vi "UMLEditor_ReadXmiFile.vi"(1 "XmiFilePath":path=path "C:/Users/Mikael/Documents/EPA/ABC.xml", 5 "error in (no error)":errorcluster) -> (15 "classInfos":T14[](array[typedef]), 16 "TypeDefs":T10[](array[typedef]), 17 "Positions":cluster{"X":i32, "Y":i32}[](array[cluster]), 19 "error out":errorcluster)   [LabVIEW 2020]
doc: "Gets current diagram values"
uses:
  <resource>/Framework/Providers/Open_GDS/UML/ReversedEngineering/ReversedEngineering ClassInfoType.ctl
  <resource>/Framework/Providers/Open_GDS/ClassProviders/Common/CommonVIs/CommonVIs_VisibilityType.ctl
  <resource>/Framework/Providers/Open_GDS/ClassProviders/Common/CommonVIs/CommonVIs_AttributeInfoType.ctl
  <resource>/Framework/Providers/Open_GDS/ClassProviders/Common/CommonVIs/CommonVIs_AttributeDataType.ctl
  <resource>/Framework/Providers/Open_GDS/UML/ReversedEngineering/ReversedEngineering_ClassDependencyDetailsType.ctl
  <resource>/Framework/Providers/Open_GDS/ClassProviders/Common/ScriptingFunctions/SubVIs/Scripting_ViDependencyType.ctl
  <resource>/Framework/Providers/Open_GDS/UML/ReversedEngineering/ReversedEngineering TypeDefType.ctl
  <resource>/Framework/Providers/Open_GDS/UML/UMLEditor/UMLEditor_ReadXmiFile_Class.ctl
  <resource>/Framework/Providers/Open_GDS/UML/UMLEditor/UMLEditor_ReadXmiFile_Attribute.ctl
  <resource>/Framework/Providers/Open_GDS/UML/UMLEditor/UMLEditor_ReadXmiFile_Method.ctl
  <resource>/Framework/Providers/Open_GDS/UML/UMLEditor/UMLEditor_ReadXmiFile_DataTypes.ctl
  <resource>/Framework/Providers/Open_GDS/UML/UMLEditor/UMLEditor_ReadXmiFile_Association.ctl
  <resource>/Framework/Providers/Open_GDS/UML/UMLEditor/UMLEditor_ReadXmiFile_AssType.ctl
  <resource>/Framework/Providers/Open_GDS/UML/UMLEditor/UMLEditor_ReadXmiFile_Generalization.ctl
  <resource>/Framework/Providers/Open_GDS/UML/UMLEditor/UMLEditor_ReadXmiFile_Links.ctl
  <resource>/Framework/Providers/Open_GDS/UML/UMLEditor/UMLEditor_ReadXmiFile_LinkType.ctl
  <resource>/Framework/Providers/Open_GDS/ClassProviders/Common/CommonVIs/CommonVIs_ClassNamePathType.ctl
panel:
  out "ClassLinks":cluster{T1[]}[](array[cluster])
  out "ClassInheritance":cluster{"Genarilization":T3[]}[](array[cluster])
  out "Associations":T4[](array[typedef])
  out "Types":T6[](array[typedef])=[{"ID"="EAJava_float", "Name"="float"}, {"ID"="EAID_9D25F9E0_C95B_4aa1_AC76_B051C1862941", "Name"="A"}, {"ID"="EAID_C3DA8127_A723_4109_B2F4_88FBFDB77E9A", "Name"="C"}]
  out "ClassMethods":cluster{T7[]}[](array[cluster])=[{[{"ID"="EAID_5C196C86_2F09_4642_AF82_8C0E9349B8CC", "Name"="M1", "Visibility"=enum."public"}]}, {[{"ID"="EAID_F6ADC8AA_458B_42d5_92A7_EFF47D20A323", "Name"="M11", "Visibility"=enum."public"}]}, {[]}]
  out "ClassAttributes":cluster{T8[]}[](array[cluster])=[{[{"ID"="EAID_78A0901B_D286_47e2_BF0A_CBA2A3759587", "Name"="Att1", "Visibility"=enum."private", "RefIdType"="EAJava_float", "AssRefId"=""}]}, {[{"ID"="EAID_dst816E9D_1FF1_4b60_8E7A_E0ACE5709CF7", "Name"="", "Visibility"=enum."public", "RefIdType"="EAID_9D25F9E0_C95B_4aa1_AC76_B051C1862941", "AssRefId"="EAID_A6816E9D_1FF1_4b60_8E7A_E0ACE5709CF7"}, {"ID"="EAID_dst1490FC_8515_4843_A058_F8B338EB0930", "Name"="", "Visibility"=enum."public", "RefIdType"="EAID_C3DA8127_A723_4109_B2F4_88FBFDB77E9A", "AssRefId"="EAID_DE1490FC_8515_4843_A058_F8B338EB0930"}]}, {[]}]
  out "Classes":T9[](array[typedef])=[{"ID"="EAID_9D25F9E0_C95B_4aa1_AC76_B051C1862941", "Name"="A", "Visibility"=enum."public", "Stereotype"="", "Description"="", "X"=0, "Y"=0}, {"ID"="EAID_C026E737_BCF9_4d6d_B726_90C39C0C8268", "Name"="B", "Visibility"=enum."public", "Stereotype"="", "Description"="", "X"=0, "Y"=0}, {"ID"="EAID_C3DA8127_A723_4109_B2F4_88FBFDB77E9A", "Name"="C", "Visibility"=enum."public", "Stereotype"="", "Description"="", "X"=0, "Y"=0}]
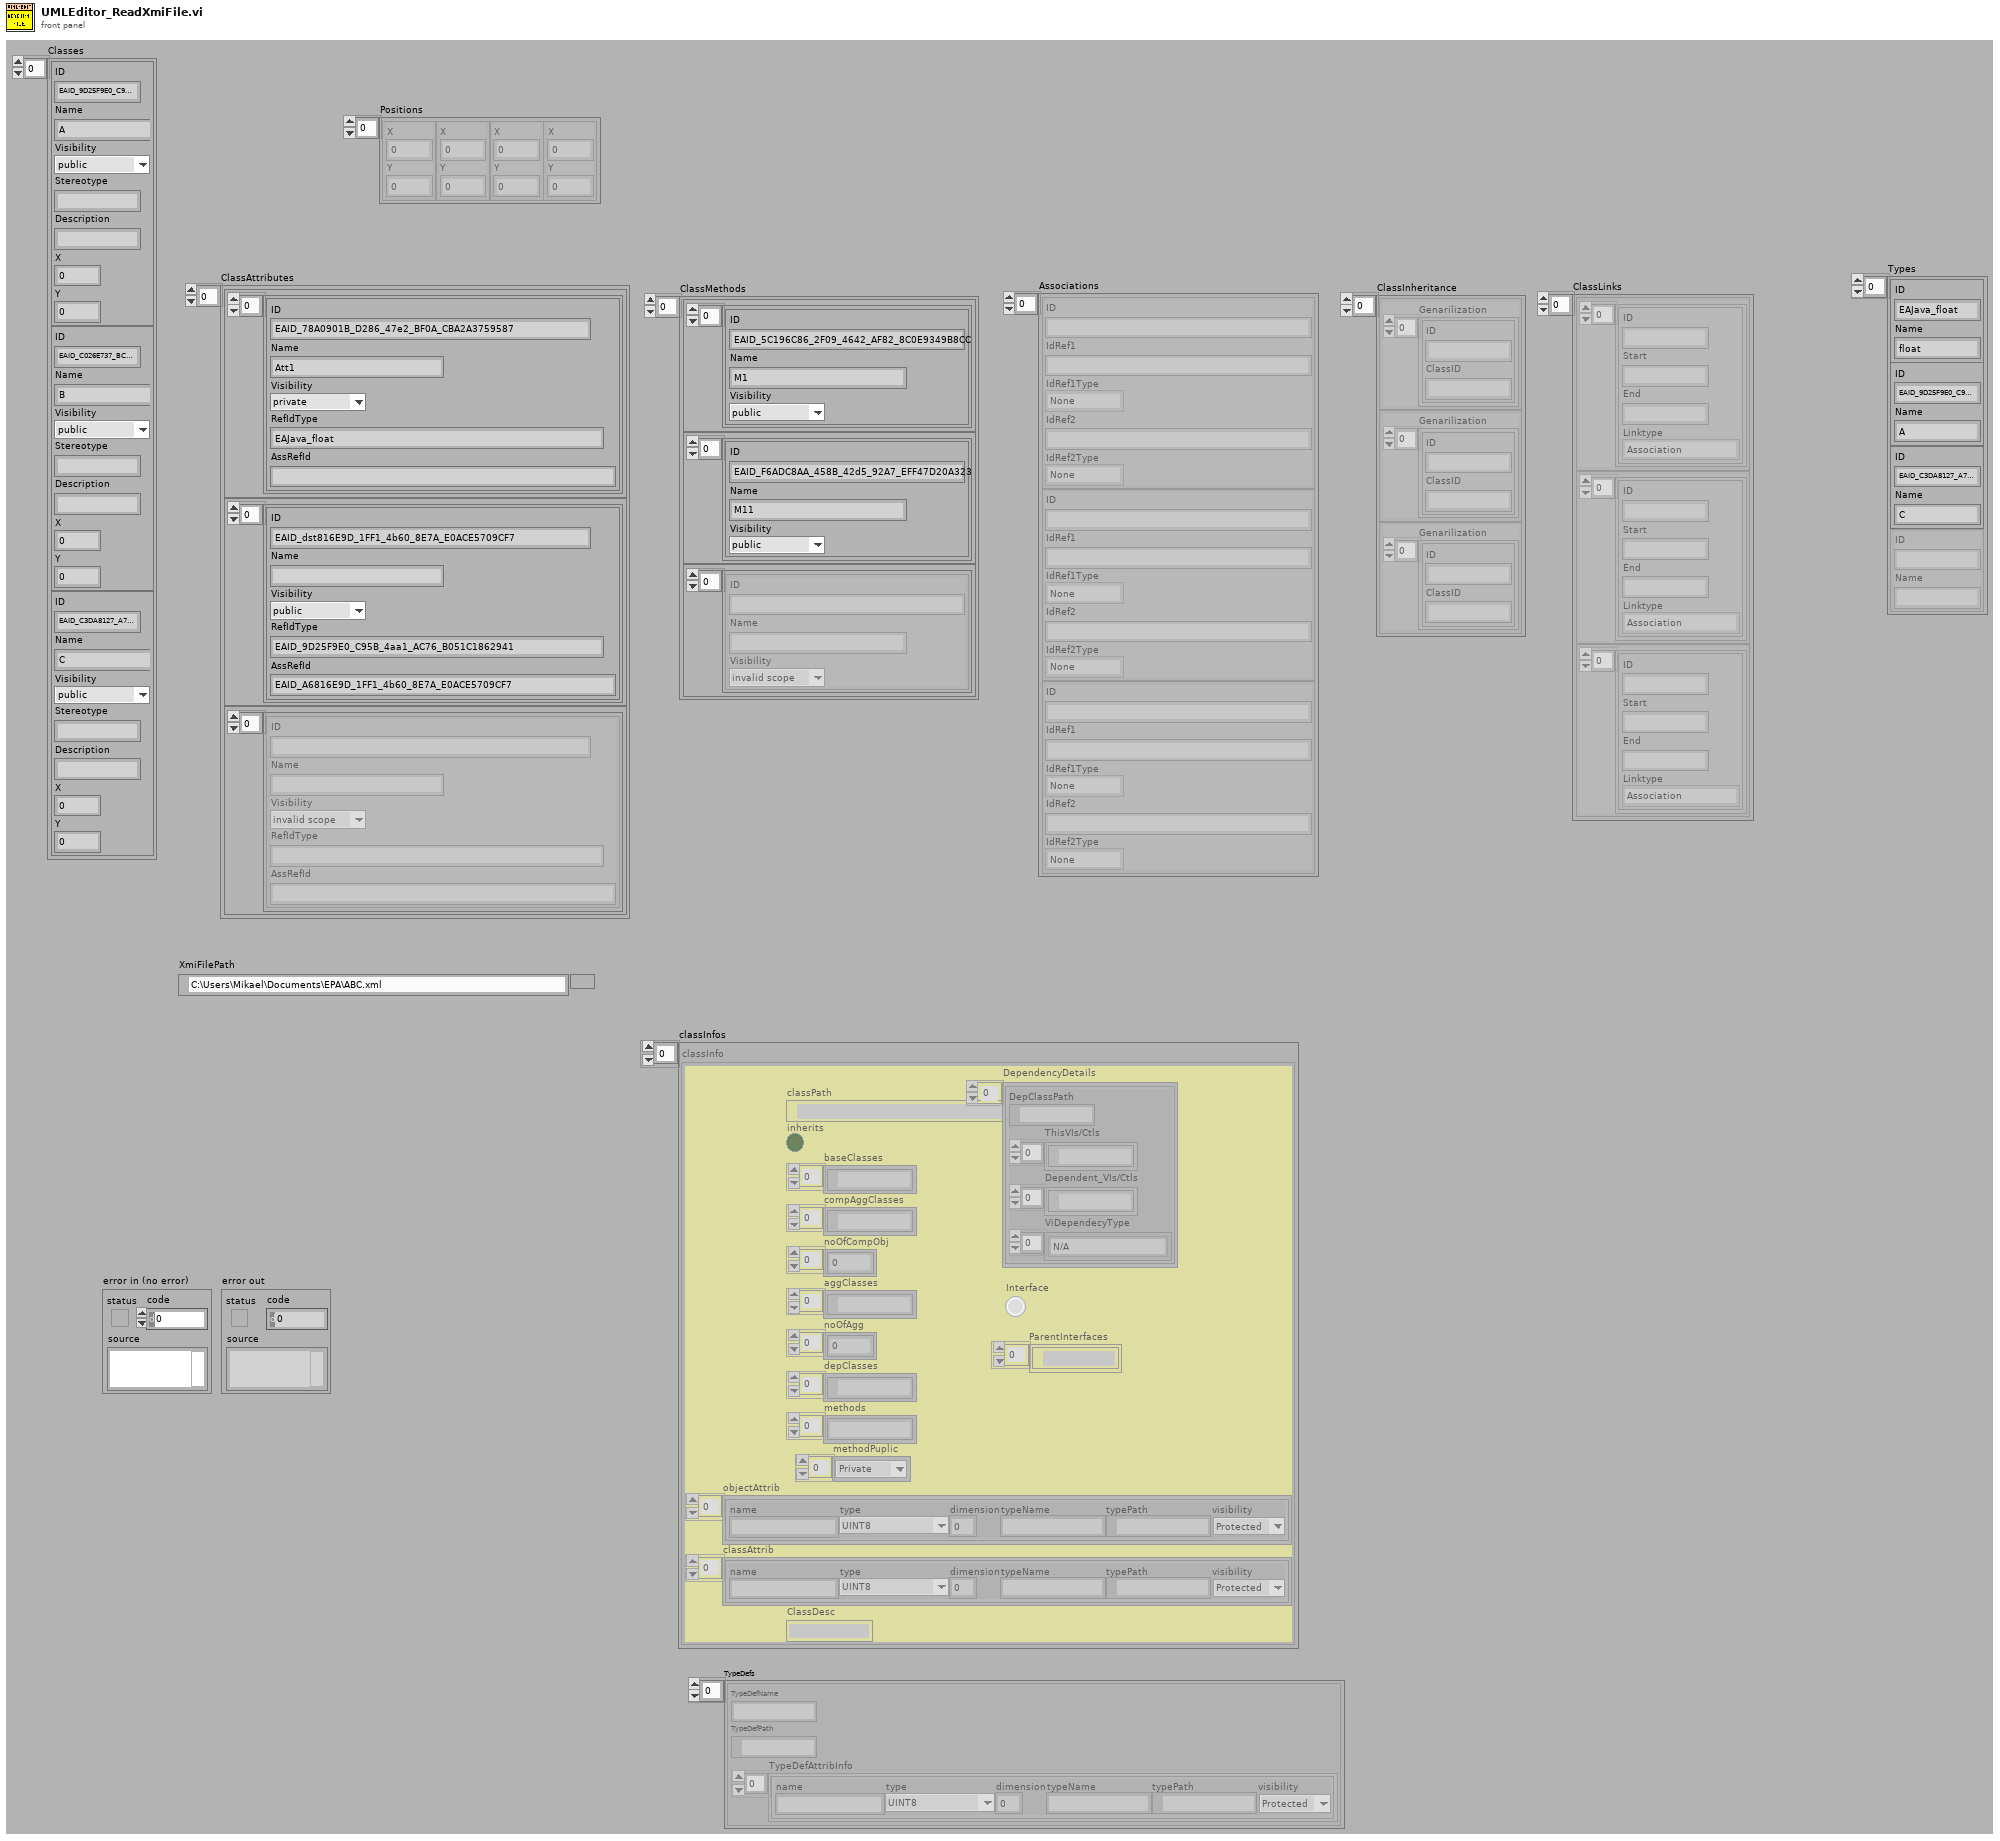
[diagram p1: front panel]
types:
  T1 = typedef "UMLEditor_ReadXmiFile_Links.ctl" = cluster{"ID":string, "Start":string, "End":string, "Linktype":T2}
  T2 = typedef "UMLEditor_ReadXmiFile_LinkType.ctl" = enum16{"Association", "Aggregation", "Generalization"}
  T3 = typedef "UMLEditor_ReadXmiFile_Generalization.ctl" = cluster{"ID":string, "ClassID":string}
  T4 = typedef "UMLEditor_ReadXmiFile_Association.ctl" = cluster{"ID":string, "IdRef1":string, "IdRef1Type":T5, "IdRef2":string, "IdRef2Type":T5}
  T5 = typedef "UMLEditor_ReadXmiFile_AssType.ctl" = enum16{"None", "Shared", "Composite"}
  T6 = typedef "UMLEditor_ReadXmiFile_DataTypes.ctl" = cluster{"ID":string, "Name":string}
  T7 = typedef "UMLEditor_ReadXmiFile_Method.ctl" = cluster{"ID":string, "Name":string, "Visibility":enum32{"invalid scope", "public", "private", "protected", "community"}}
  T8 = typedef "UMLEditor_ReadXmiFile_Attribute.ctl" = cluster{"ID":string, "Name":string, "Visibility":enum32{"invalid scope", "public", "private", "protected", "community"}, "RefIdType":string, "AssRefId":string}
  T9 = typedef "UMLEditor_ReadXmiFile_Class.ctl" = cluster{"ID":string, "Name":string, "Visibility":enum32{"invalid scope", "public", "private", "protected", "community"}, "Stereotype":string, "Description":string, "X":i32, "Y":i32}
  T10 = typedef "ReversedEngineering TypeDefType.ctl" = cluster{"TypeDefName":string, "TypeDefPath":path, "TypeDefAttribInfo":T11[]}
  T11 = typedef "CommonVIs_AttributeInfoType.ctl" = cluster{"name":string, "type":T12, "dimension":i32, "typeName":string, "typePath":path, "visibility":T13}
  T12 = typedef "CommonVIs_AttributeDataType.ctl" = enum16{"UINT8", "INT8", "UINT16", "INT16", "UINT32", "INT32", "UINT64", "INT64", "SGL", "DBL", "EXT", "CSG", "CDB", "CXT", "TimeStamp", "STRING", "PATH", "BOOL", "ENUM", "RefNum", "VIRefNum", "LabVIEW Class", "Cluster", "Variant", "TypeDef", "Waveform", "LabVIEW Object", "Other", "void", "Set", "Map"}
  T13 = typedef "CommonVIs_VisibilityType.ctl" = enum16{"Public", "Private", "Protected"}
  T14 = typedef "ReversedEngineering ClassInfoType.ctl" = cluster{"classPath":path, "inherits":bool, "baseClasses":path[], "compAggClasses":path[], "noOfCompObj":i32[], "aggClasses":path[], "noOfAgg":i32[], "depClasses":path[], "methods":string[], "methodPuplic":T13[], "objectAttrib":T11[], "classAttrib":T11[], "ClassDesc":string, "DependencyDetails":T15[], "Interface":bool, "ParentInterfaces":path[]}
  T15 = typedef "ReversedEngineering_ClassDependencyDetailsType.ctl" = cluster{"DepClassPath":path, "ThisVIs/Ctls":path[], "Dependent_VIs/Ctls":path[], "ViDependecyType":T16[]}
  T16 = typedef "Scripting_ViDependencyType.ctl" = enum16{"N/A", "Launches"}
  T17 = cluster{"dependencyClassPath":path[], "topVIPath":path, "classInfos":T14[], "calleesVIs":path[], "VIRef":refnum<vi>[], "TypeDefs":T10[], "TopVIPath":path, "SearchOnlyClasses":bool, "SearchDirs":path[], "SearchOnlyTopVIs":bool, "lvclasses":path[], "Classes":T9[], "ClasseStrings":string[], "ClassAttributes":cluster{T8[]}[], "ClassMethods":cluster{T7[]}[], "text":string, "Types":T6[], "ClassInheritance":cluster{"Genarilization":T3[]}[], "Associations":T4[], "Positions":cluster{"X":i32, "Y":i32}[], "ClassLinks":cluster{T1[]}[]}
  T18 = enum32{"invalid scope", "public", "private", "protected", "community"}
  T19 = typedef "CommonVIs_ClassNamePathType.ctl" = cluster{"ClassNamn":string, "ClassPath":path, "InterfaceClass":bool}
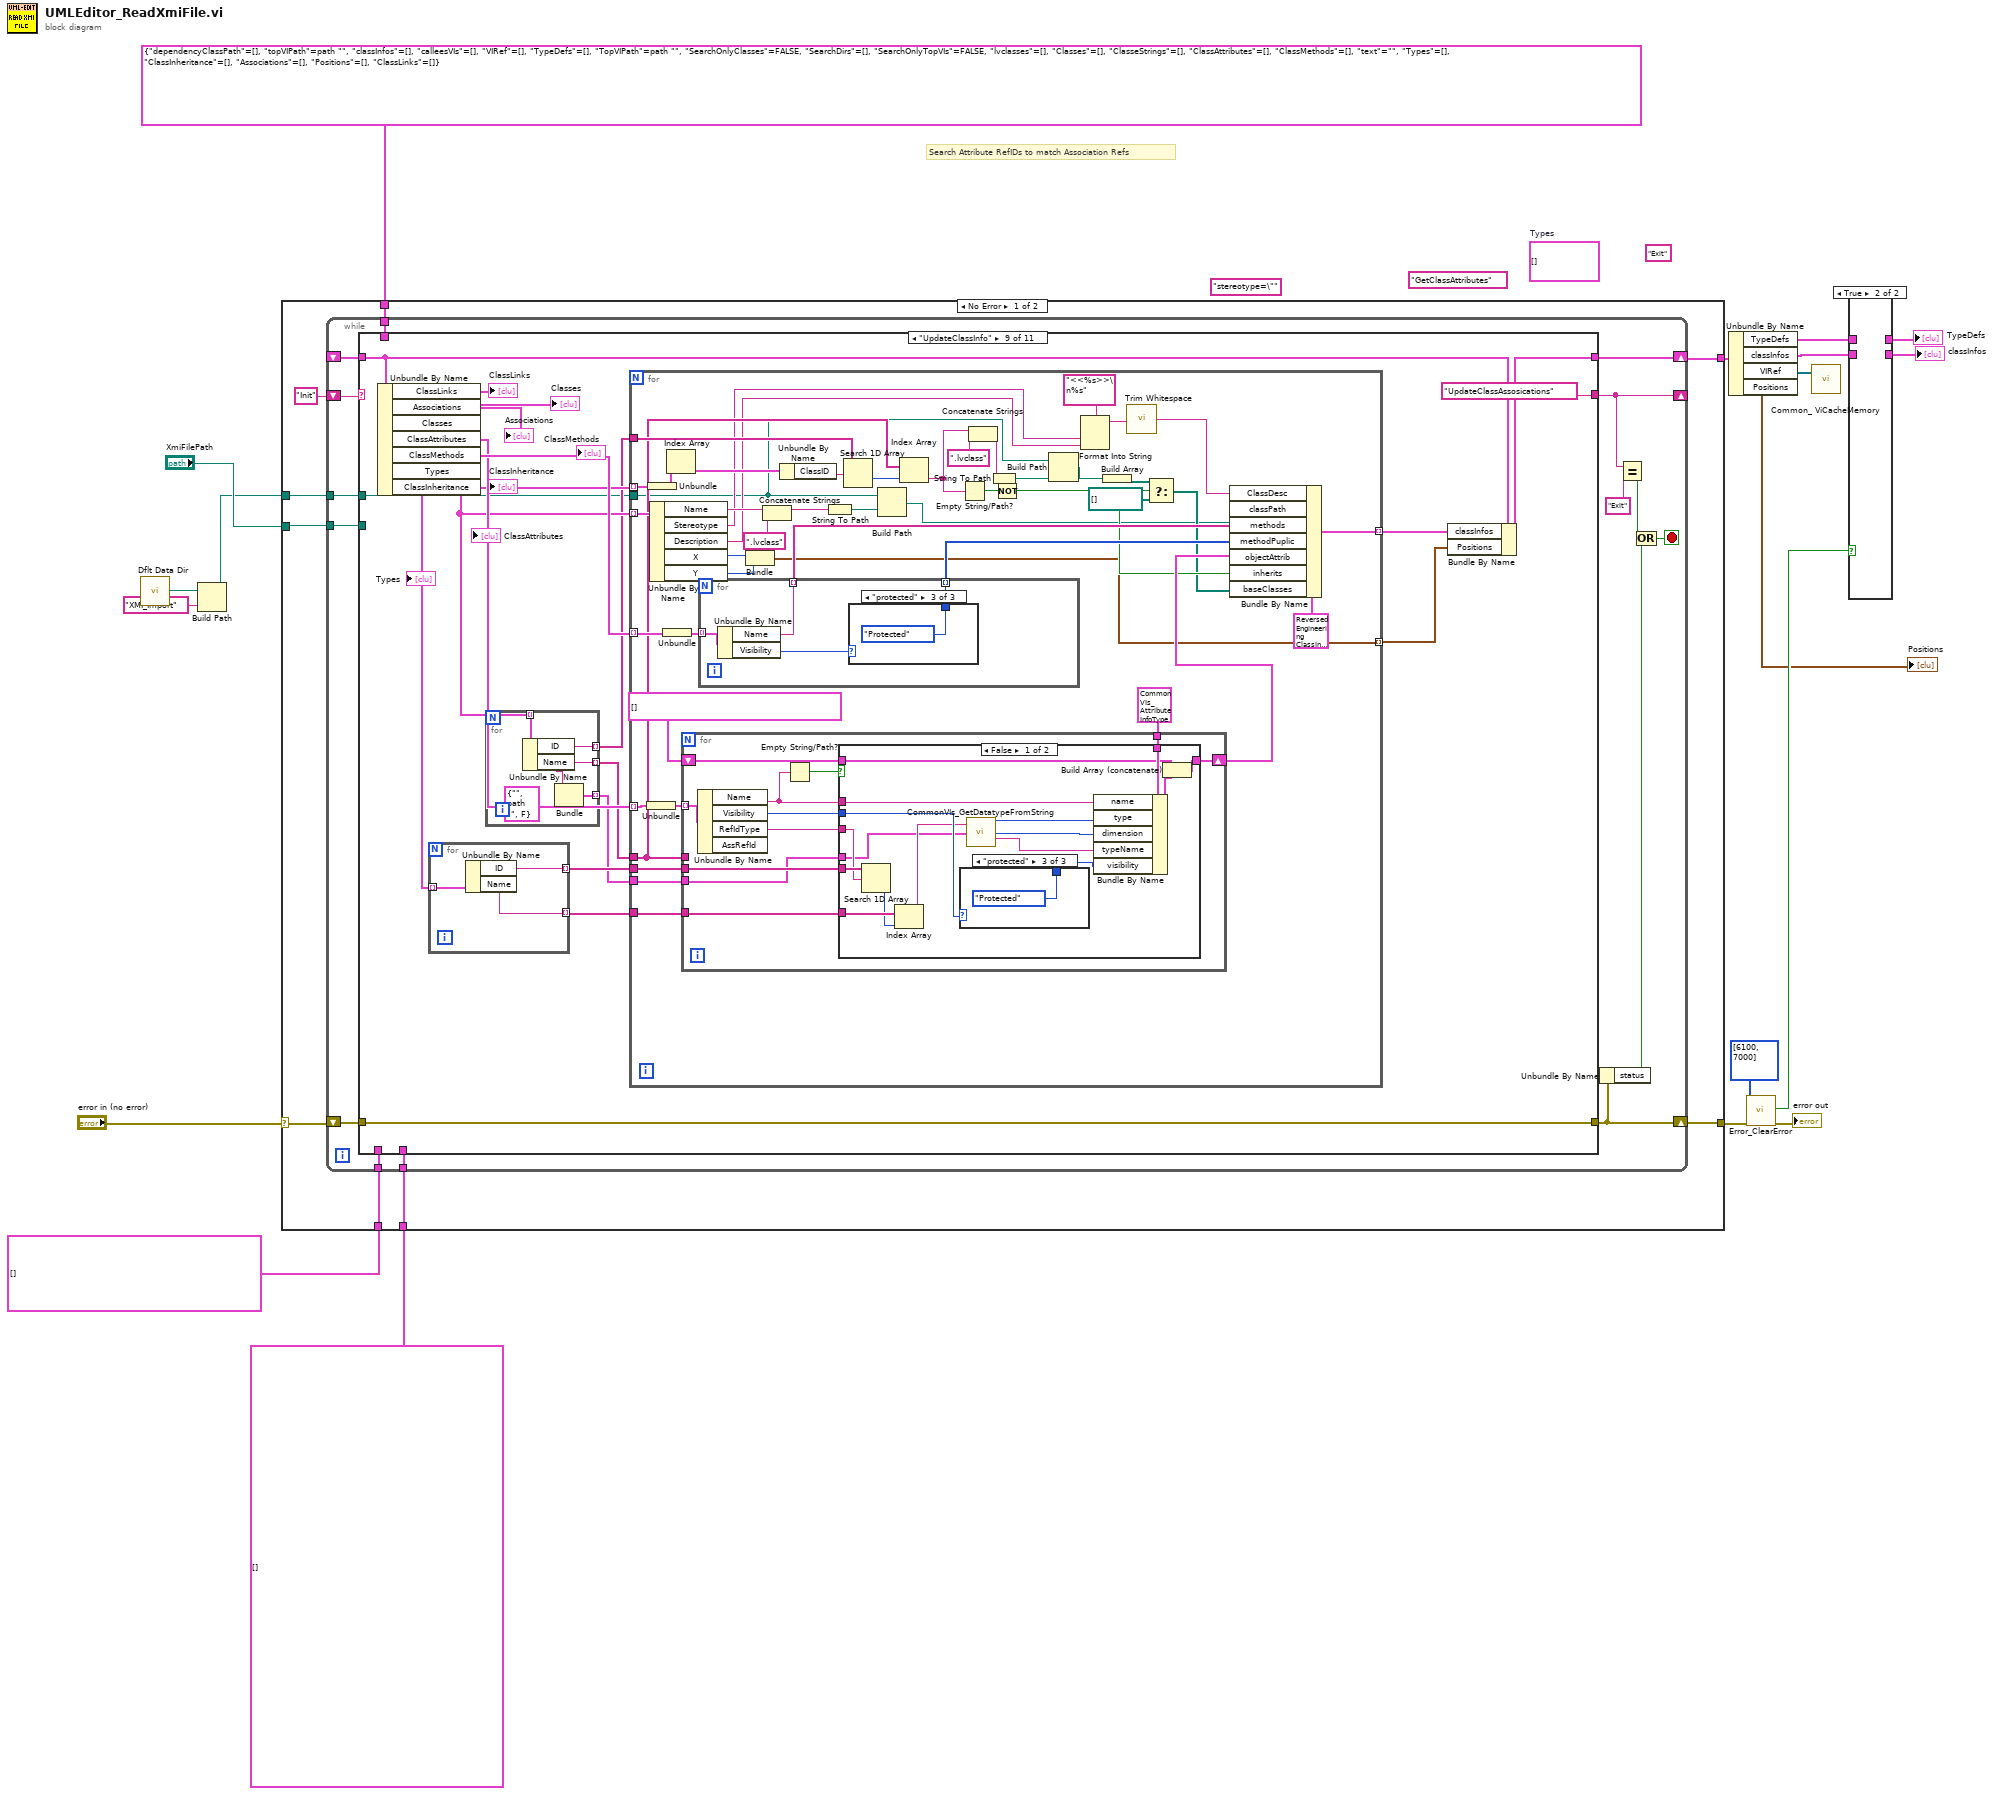
[diagram p0: block diagram]
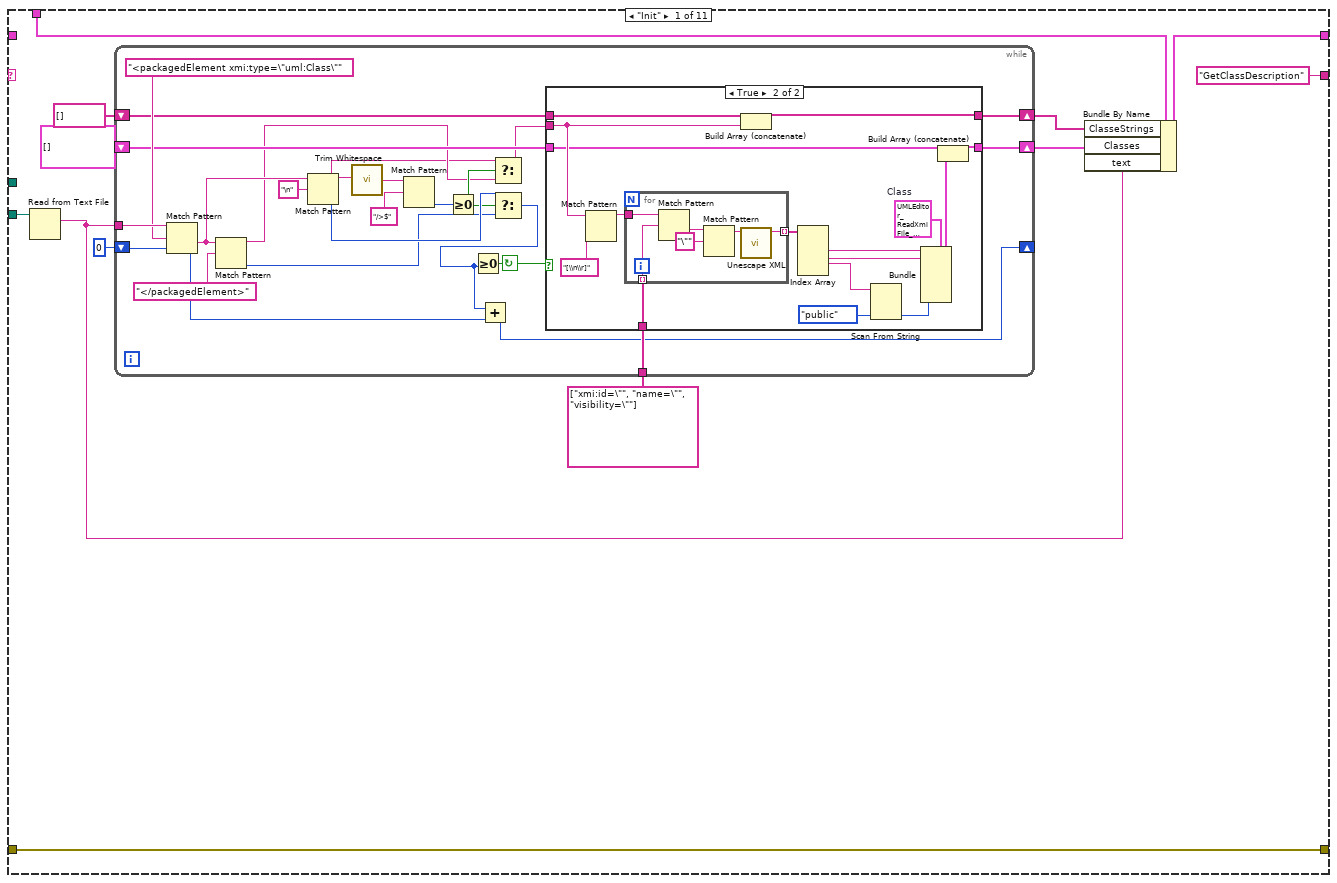
[diagram p3: hidden frame]
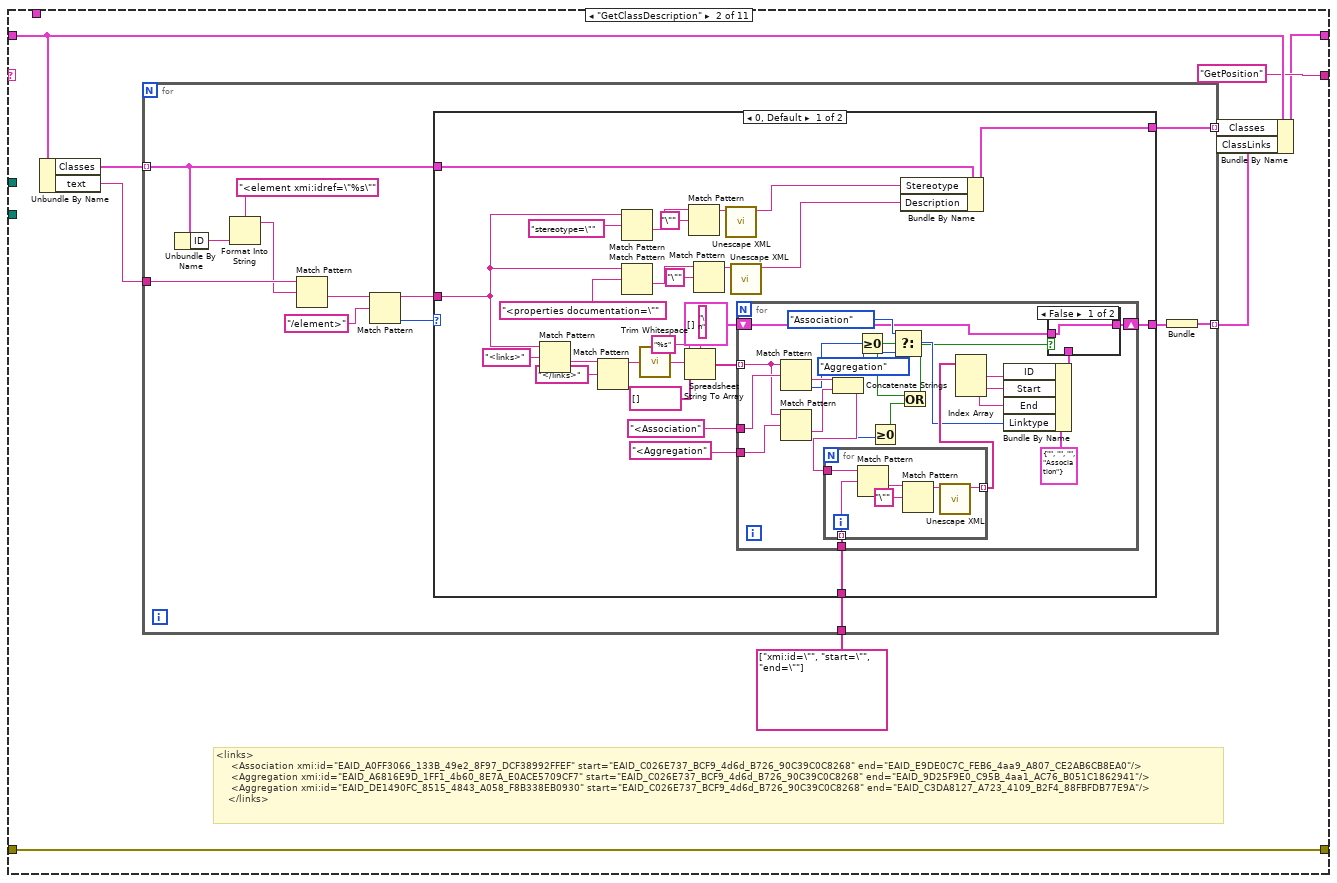
[diagram p5: hidden frame]
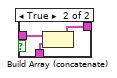
[diagram p6: hidden frame]
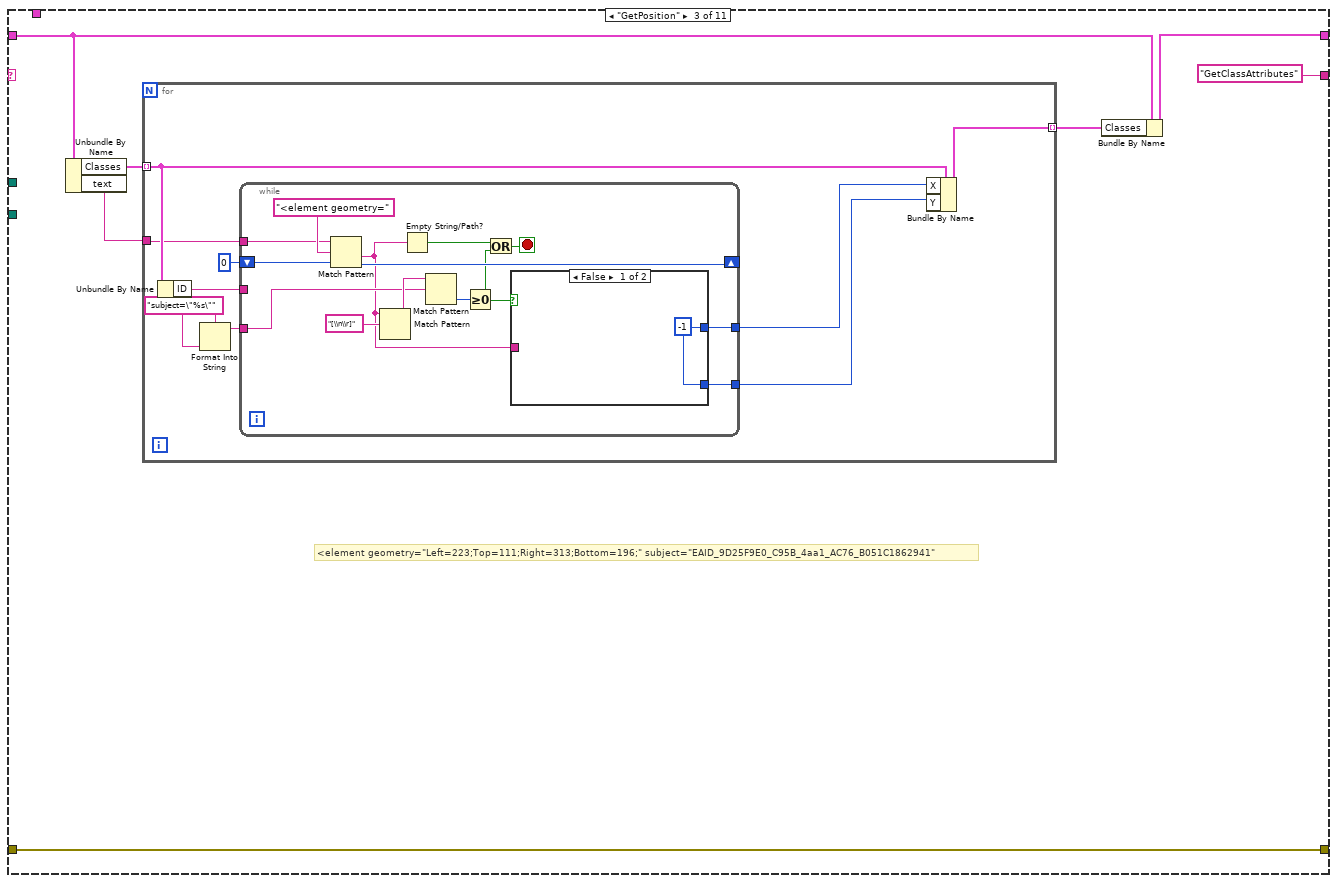
[diagram p8: hidden frame]
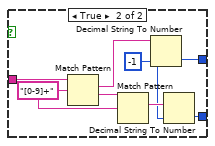
[diagram p9: hidden frame]
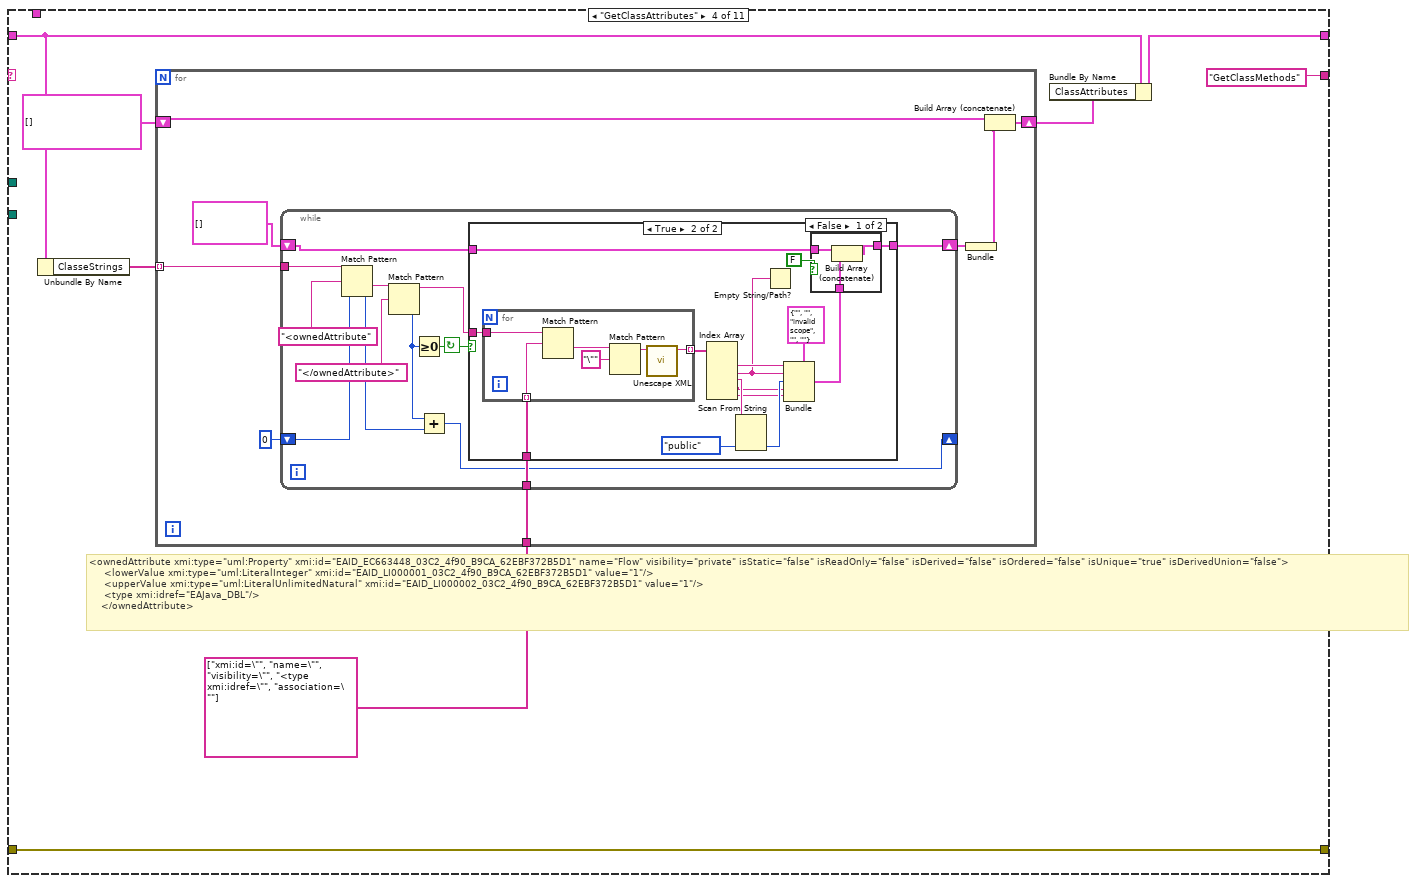
[diagram p10: hidden frame]
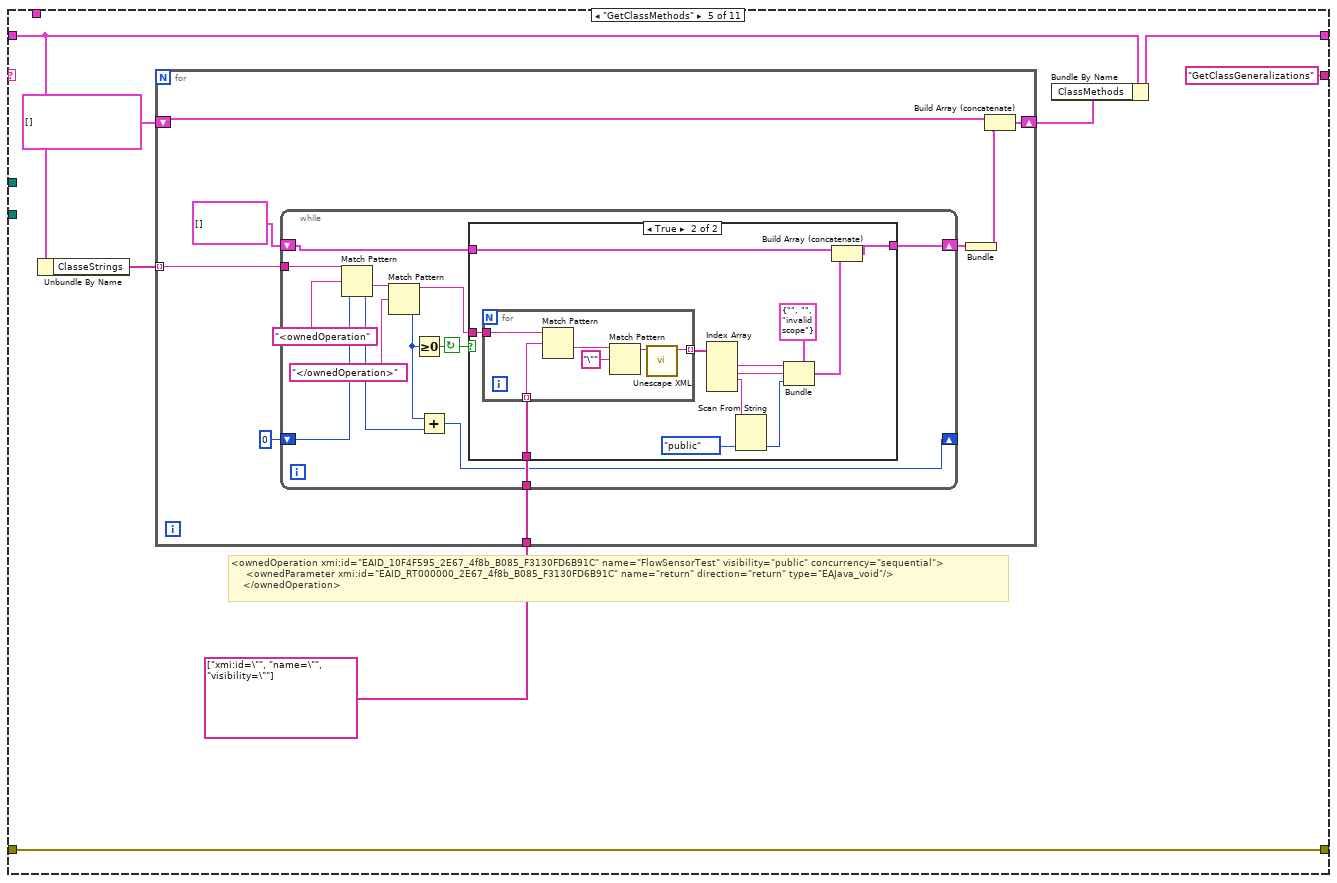
[diagram p13: hidden frame]
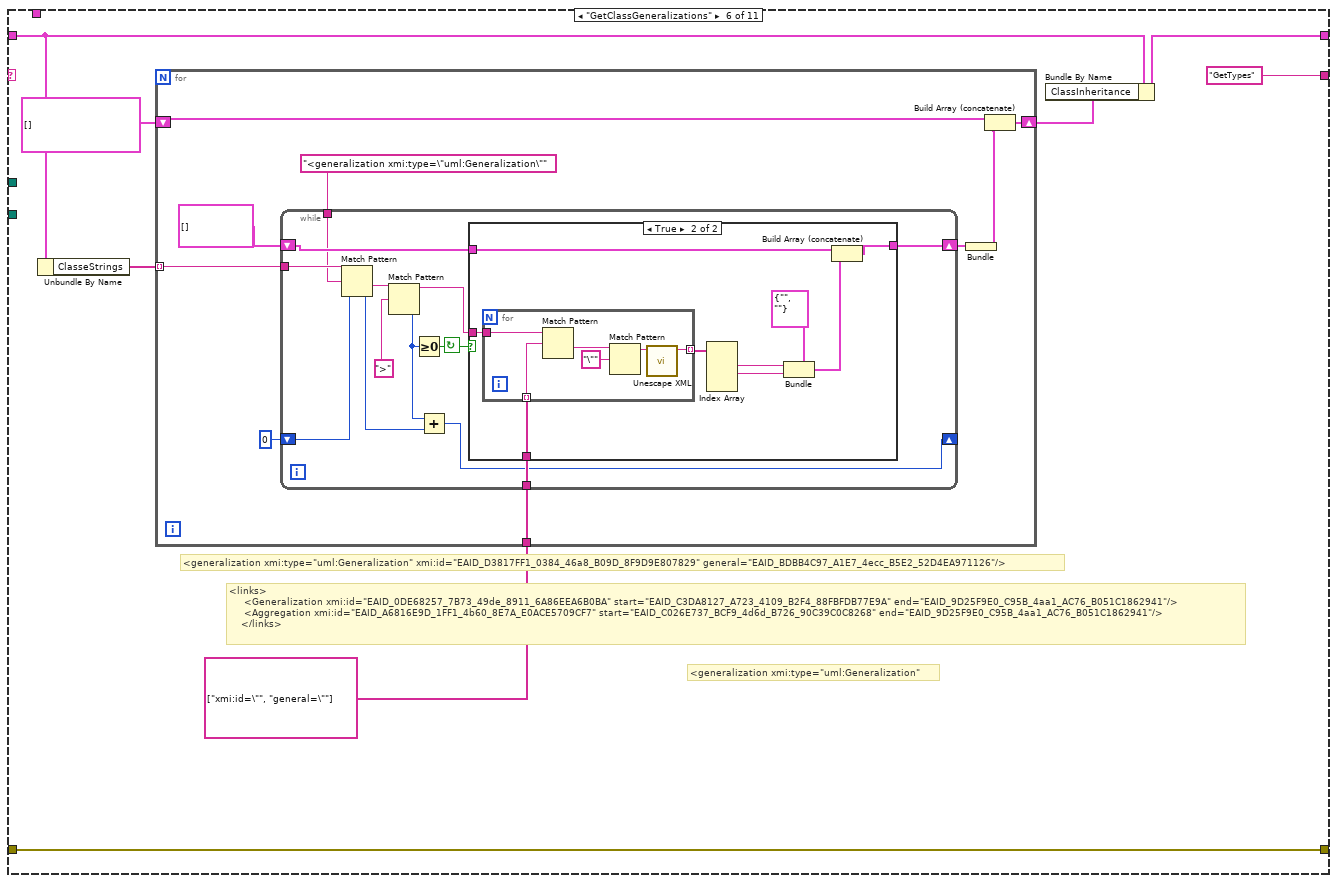
[diagram p15: hidden frame]
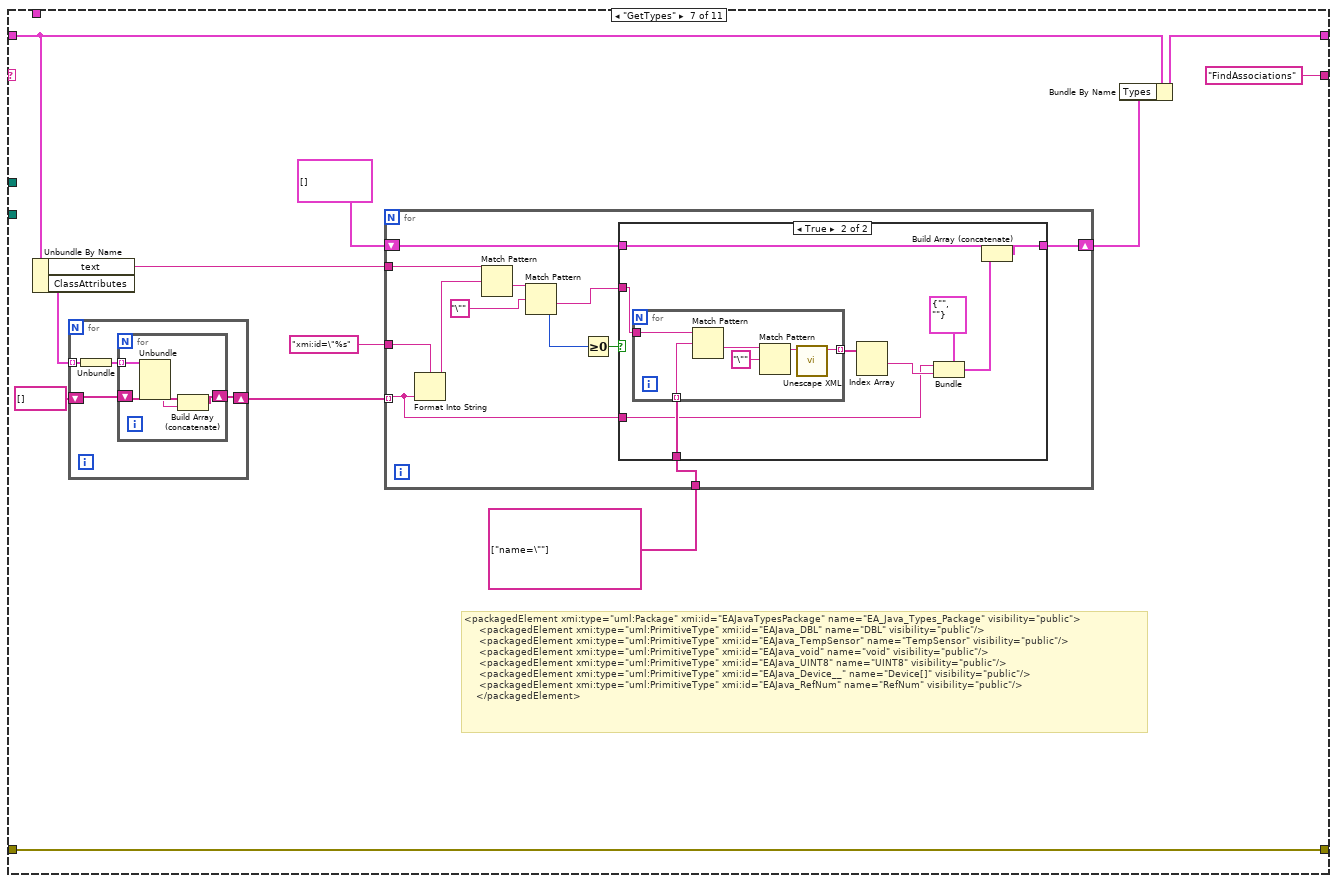
[diagram p17: hidden frame]
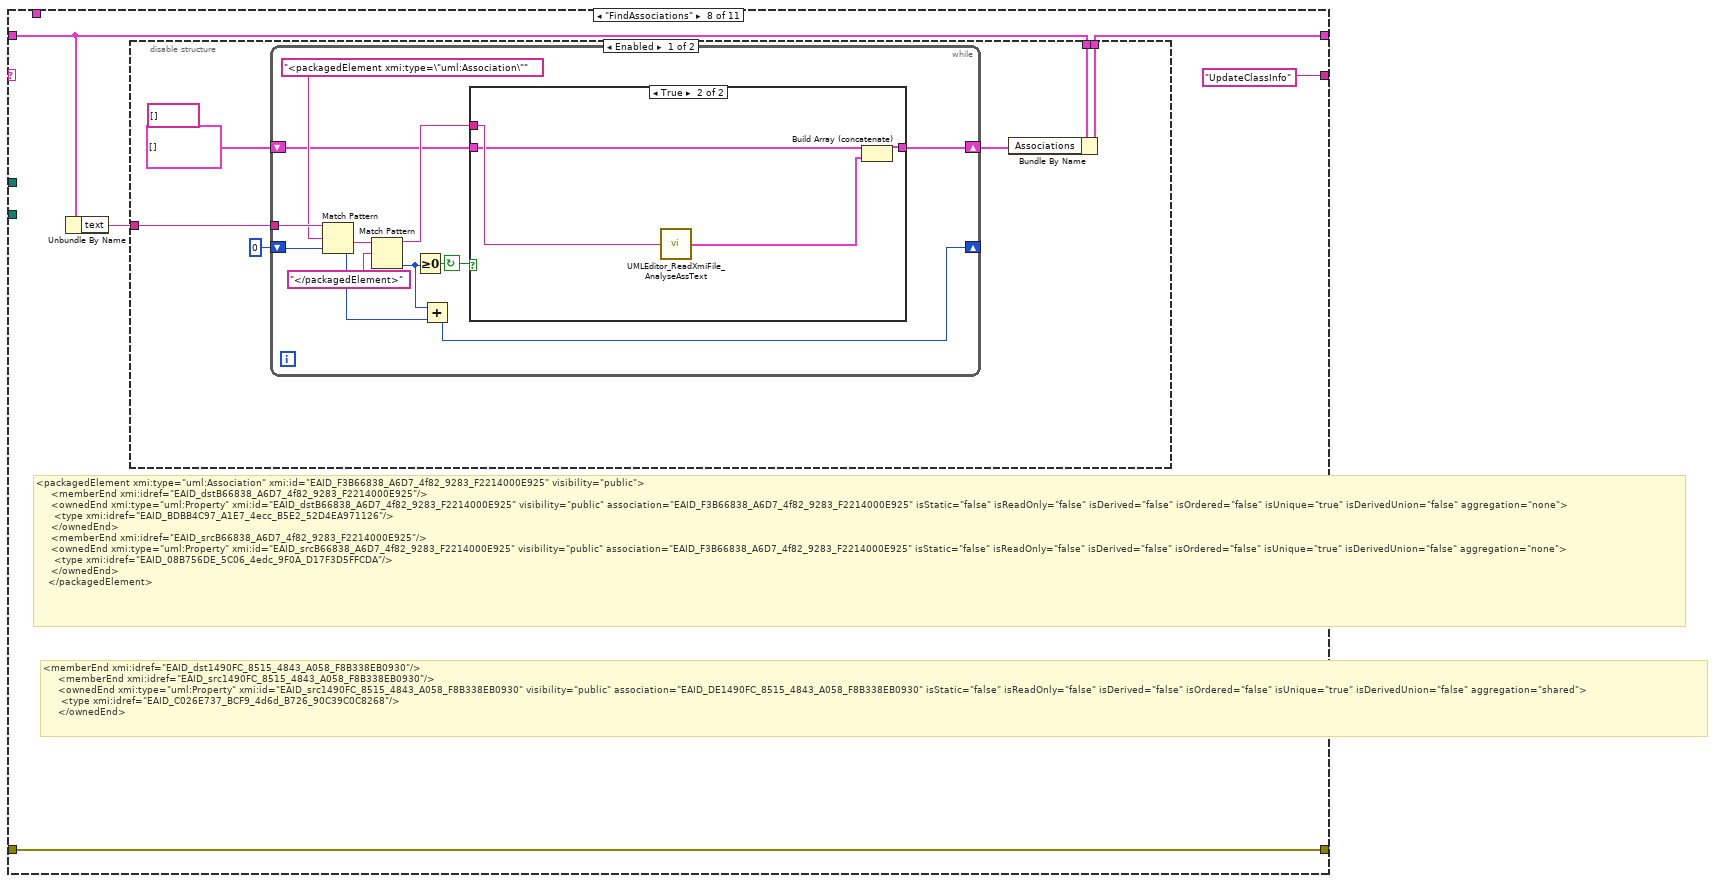
[diagram p19: hidden frame]
diagram:
  (unwired) "Exit" ("y")
  (unwired) "GetClassAttributes"
  (unwired) "stereotype=\""
  (unwired) T6[] []  # Types
  # "Search Attribute RefIDs to match Association Refs"
  n1 = call <vilib>:"Dflt Data Dir.vi"() -> ("App:Default Data Directory"=w3:path)
  n2 = Build Path(base path=w3, name or relative path="XMI_Import") -> (appended path=w1:path)
  n3 = case shown="No Error" "error in (no error)" {
    selector: "error in (no error)" -> [w27 w747]
    tunnel: [w26 w747] -> w16
    tunnel: [w25 _] -> w18
    tunnel: T17 {"dependencyClassPath"=[], "topVIPath"=path "", "classInfos"=[], "calleesVIs"=[], "VIRef"=[], "TypeDefs"=[], "TopVIPath"=path "", "SearchOnlyClasses"=FALSE, "SearchDirs"=[], "SearchOnlyTopVIs"=FALSE, "lvclasses"=[], "Classes"=[], "ClasseStrings"=[], "ClassAttributes"=[], "ClassMethods"=[], "text"="", "Types"=[], "ClassInheritance"=[], "Associations"=[], "Positions"=[], "ClassLinks"=[]} ("Cluster") -> [w24 _]
    tunnel: T14[] [] -> [w23 _]
    tunnel: T10[] [] -> [w22 _]
    tunnel: "XmiFilePath" -> [w21 _]
    tunnel: w1 -> [w20 _]
    frame No Error {
      n4 = while {
        shift-right: [w40] -> _
        shift-left: "Init" -> [w43]
        shift-right: [w41] -> w26
        shift-left: w27 -> [w42]
        shift-right: [w34] -> w25
        shift-left: _ -> [w35]
        tunnel: w24 -> [w33]
        tunnel: w23 -> [w32]
        tunnel: w22 -> [w31]
        tunnel: w21 -> [w30]
        tunnel: w20 -> [w29]
        stop <- w36 stop-if-true
        n5 = case shown="\"UpdateClassInfo\"" w43 {
          tunnel: w42 -> [w55 w106 w187 w227 w281 w329 w375 w427 w469 w568 w744]
          tunnel: [w55 w106 w187 w227 w281 w329 w375 w427 w469 w568 w744] -> w41
          tunnel: ["GetClassDescription" "GetPosition" "GetClassAttributes" "GetClassMethods" "GetClassGeneralizations" "GetTypes" "FindAssociations" "UpdateClassInfo" "UpdateClassAssosications" ("y") "Exit" ("y") "Exit" ("y")] -> w40
          tunnel: w35 -> [_ w111 w192 w230 w285 w333 w384 w423 w461 w564 w746]
          tunnel: [w46 w109 w190 w228 w283 w331 w383 w426 w460 w575 w746] -> w34
          tunnel: w33 -> [w47 _ _ _ _ _ _ _ _ _ _]
          tunnel: w32 -> [_ _ _ _ _ _ _ _ _ _ _]
          tunnel: w31 -> [_ _ _ _ _ _ _ _ _ _ _]
          tunnel: w30 -> [w54 _ _ _ _ _ _ _ _ _ _]
          tunnel: w29 -> [_ _ _ _ _ _ _ _ w454 w569 _]
          frame "Init" {
            n6 = Read from Text File(file (use dialog)=w54) -> (text=w45:string)  [unwired: 3 in, 3 out]
            n7 = while {
              tunnel: w45 -> [w79]
              shift-right: [w75] -> w48
              shift-left: string[] [] -> [w76]
              shift-right: [w68] -> _
              shift-left: 0 ("offset past match") -> [w73]
              tunnel: string[] ["xmi:id=\"", "name=\"", "visibility=\""] -> [w72]
              shift-right: [w71] -> w49
              shift-left: T9[] [] -> [w70]
              stop <- w74 continue-if-true
              n8 = Match Pattern(string=w79, regular expression="<packagedElement xmi:type=\"uml:Class\"", offset (0)=w73) -> (after substring=w62:string, offset past match=w69:i32)  [unwired: 2 out]
              n9 = Match Pattern(string=w62, regular expression="</packagedElement>") -> (before substring=w58:string, offset past match=w60:i32)  [unwired: 1 in, 2 out]
              n10 = Match Pattern(string=w62, regular expression="\n") -> (before substring=w57:string, offset past match=w67:i32)  [unwired: 1 in, 2 out]
              n11 = call <vilib>:"Trim Whitespace.vi"("string"=w57) -> ("trimmed string"=w64:string)  [unwired: 1 in]
              n12 = Match Pattern(string=w64, regular expression="/>$") -> (offset past match=w66:i32)  [unwired: 1 in, 3 out]
              n13 = Greater Or Equal To 0?(x=w66) -> (x >= 0?=w59:bool)
              n14 = Select(t=w57, s=w59, f=w58) -> (s? t:f=w56:string)
              n15 = Select(t=w67, s=w59, f=w60) -> (s? t:f=w61:i32)
              n16 = Greater Or Equal To 0?(x=w61) -> (x >= 0?=w74:bool)
              n17 = Add(x=w61, y=w69) -> (x+y=w68:i32)
              n18 = case shown="True" w74 {
                tunnel: w76 -> [w81 w97]
                tunnel: [w81 w96] -> w75
                tunnel: w56 -> [_ w95]
                tunnel: w72 -> [_ w93]
                tunnel: w70 -> [w80 w83]
                tunnel: [w80 w84] -> w71
                frame False {
                }
                frame True {
                  w90 = T9 {"ID"="", "Name"="", "Visibility"=enum."invalid scope", "Stereotype"="", "Description"="", "X"=0, "Y"=0}  # Class
                  n19 = Match Pattern(string=w95, regular expression="[\\n\\r]") -> (before substring=w92:string)  [unwired: 1 in, 3 out]
                  n20 = for {
                    tunnel: w93 -> [w103] mode=indexing
                    tunnel: w92 -> [w102]
                    tunnel: [w98] -> w91 mode=indexing
                    n21 = Match Pattern(string=w102, regular expression=w103) -> (after substring=w101:string)  [unwired: 1 in, 3 out]
                    n22 = Match Pattern(string=w101, regular expression="\"") -> (before substring=w99:string)  [unwired: 1 in, 3 out]
                    n23 = call <vilib>:"Unescape XML.vi"("XML String In"=w99) -> ("XML String Out"=w98:string)  [unwired: 9 in, 1 out]
                  }
                  n24 = Build Array (concatenate)(w97, w95) -> (w96:string[])
                  n25 = Index Array(array=w91) -> (element #1=w89:string, element #2=w88:string, element #3=w87:string)  [unwired: 4 in, 1 out]
                  n26 = Scan From String(input string=w87, default 1=T18."public" ("Visibility")) -> (output 1=w86:T18)  [unwired: 3 in, 3 out]
                  n27 = Bundle(cluster=w90, "ID"=w89, "Name"=w88, "Visibility"=w86) -> (w82:T9)  [unwired: 4 in]
                  n28 = Build Array (concatenate)(w83, w82) -> (w84:T9[])
                }
              }
            }
            n29 = Bundle By Name(cluster=w47, "ClasseStrings"=w48, "Classes"=w49, "text"=w45) -> (w46:T17)
          }
          frame "GetClassDescription" {
            # "<links>\n\t\t\t\t\t<Association xmi:id=\"EAID_A0FF3066_133B_49e2_8F97_DCF38992FFEF\" start=\"EAID_C026E737_BCF9_4d6d_B726_90C39C0C8268\" end=\"EAID_E9DE0C7C_FEB6_4aa9_A807_CE2AB6CB8EA0\"/>\n\t\t\t\t\t<Aggregation xmi:id=\"EAID_A6816E9D_1FF1_4b60_8E7A_E0ACE5709CF7\" start=\"EAID_C026E737_BCF9_4d6d_B726_90C39C0C8268\" end=\"EAID_9D25F9E0_C95B_4aa1_AC76_B051C1862941\"/>\n\t\t\t\t\t<Aggregation xmi:id=\"EAID_DE1490FC_8515_4843_A058_F8B338EB0930\" start=\"EAID_C026E737_BCF9_4d6d_B726_90C39C0C8268\" end=\"EAID_C3DA8127_A723_4109_B2F4_88FBFDB77E9A\"/>\n\t\t\t\t</links>"
            n30 = Unbundle By Name(w111) -> ("Classes"=w112:T9[], "text"=w107:string)
            n31 = for {
              tunnel: w112 -> [w123] mode=indexing
              tunnel: [w125] -> w108 mode=indexing
              tunnel: w107 -> [w121]
              tunnel: string[] ["xmi:id=\"", "start=\"", "end=\""] -> [w115]
              tunnel: [w113] -> w104 mode=indexing
              n32 = Unbundle By Name(w123) -> ("ID"=w122:string)
              n33 = Format Into String(format string="<element xmi:idref=\"%s\"", w122) -> (resulting string=w120:string)  [unwired: 2 in, 1 out]
              n34 = Match Pattern(string=w121, regular expression=w120) -> (after substring=w119:string)  [unwired: 1 in, 3 out]
              n35 = Match Pattern(string=w119, regular expression="/element>") -> (before substring=w116:string, offset past match=w117:i32)  [unwired: 1 in, 2 out]
              n36 = case shown="0, Default" w117 {
                tunnel: [w152 w186] -> w125
                tunnel: w123 -> [w151 w186]
                tunnel: w116 -> [w140 _]
                tunnel: w115 -> [w128 _]
                tunnel: [w126 _] -> w114
                frame 0, Default {
                  n37 = Match Pattern(string=w140, regular expression="<links>") -> (after substring=w138:string)  [unwired: 1 in, 3 out]
                  n38 = Match Pattern(string=w138, regular expression="</links>") -> (before substring=w136:string)  [unwired: 1 in, 3 out]
                  n39 = Match Pattern(string=w140, regular expression="stereotype=\"") -> (after substring=w142:string)  [unwired: 1 in, 3 out]
                  n40 = Match Pattern(string=w140, regular expression="<properties documentation=\"") -> (after substring=w147:string)  [unwired: 1 in, 3 out]
                  n41 = call <vilib>:"Trim Whitespace.vi"("string"=w136) -> ("trimmed string"=w135:string)  [unwired: 1 in]
                  n42 = Spreadsheet String To Array(delimiter (Tab)="\n", format string="%s", spreadsheet string=w135, array type (2D Dbl)=string[] []) -> (array=w131:string[])
                  n43 = Match Pattern(string=w142, regular expression="\"") -> (before substring=w144:string)  [unwired: 1 in, 3 out]
                  n44 = Match Pattern(string=w147, regular expression="\"") -> (before substring=w148:string)  [unwired: 1 in, 3 out]
                  n45 = call <vilib>:"Unescape XML.vi"("XML String In"=w144) -> ("XML String Out"=w141:string)  [unwired: 9 in, 1 out]
                  n46 = call <vilib>:"Unescape XML.vi"("XML String In"=w148) -> ("XML String Out"=w146:string)  [unwired: 9 in, 1 out]
                  n47 = for {
                    tunnel: w131 -> [w174] mode=indexing
                    tunnel: "<Association" ("regular expression") -> [w175]
                    tunnel: "<Aggregation" ("regular expression") -> [w173]
                    tunnel: w128 -> [w169]
                    shift-right: [w153] -> w126
                    shift-left: T1[] [] -> [w154]
                    n48 = Match Pattern(string=w174, regular expression=w175) -> (after substring=w172:string, offset past match=w167:i32)  [unwired: 1 in, 2 out]
                    n49 = Match Pattern(string=w174, regular expression=w173) -> (after substring=w171:string, offset past match=w159:i32)  [unwired: 1 in, 2 out]
                    n50 = Concatenate Strings(w172, w171) -> (w170:string)
                    n51 = for {
                      tunnel: w169 -> [w185] mode=indexing
                      tunnel: w170 -> [w184]
                      tunnel: [w180] -> w165 mode=indexing
                      n52 = Match Pattern(string=w184, regular expression=w185) -> (after substring=w183:string)  [unwired: 1 in, 3 out]
                      n53 = Match Pattern(string=w183, regular expression="\"") -> (before substring=w181:string)  [unwired: 1 in, 3 out]
                      n54 = call <vilib>:"Unescape XML.vi"("XML String In"=w181) -> ("XML String Out"=w180:string)  [unwired: 9 in, 1 out]
                    }
                    n55 = Greater Or Equal To 0?(x=w167) -> (x >= 0?=w157:bool)
                    n56 = Greater Or Equal To 0?(x=w159) -> (x >= 0?=w158:bool)
                    n57 = Select(t=UMLEditor_ReadXmiFile_LinkType."Association" ("Linktype"), s=w157, f=UMLEditor_ReadXmiFile_LinkType."Aggregation" ("Linktype")) -> (s? t:f=w161:T2)
                    n58 = Or(x=w157, y=w158) -> (x .or. y?=w156:bool)
                    n59 = Index Array(array=w165) -> (element #1=w164:string, element #2=w163:string, element #3=w162:string)  [unwired: 3 in]
                    n60 = Bundle By Name(cluster=T1 {"ID"="", "Start"="", "End"="", "Linktype"=enum."Association"} ("Association"), "ID"=w164, "Start"=w163, "End"=w162, "Linktype"=w161) -> (w155:T1)
                    n61 = case shown="False" w156 {
                      tunnel: w155 -> [_ w179]
                      tunnel: w154 -> [w176 w178]
                      tunnel: [w176 w177] -> w153
                      frame False {
                      }
                      frame True {
                        n62 = Build Array (concatenate)(w178, w179) -> (w177:T1[])
                      }
                    }
                  }
                  n63 = Bundle By Name(cluster=w151, "Stereotype"=w141, "Description"=w146) -> (w152:T9)
                }
                frame -1 {
                }
              }
              n64 = Bundle(w114) -> (w113:cluster{T1[]})  [unwired: 1 in]
            }
            n65 = Bundle By Name(cluster=w111, "Classes"=w108, "ClassLinks"=w104) -> (w109:T17)
          }
          frame "GetPosition" {
            # "<element geometry=\"Left=223;Top=111;Right=313;Bottom=196;\" subject=\"EAID_9D25F9E0_C95B_4aa1_AC76_B051C1862941\""
            n66 = Unbundle By Name(w192) -> ("Classes"=w193:T9[], "text"=w188:string)
            n67 = for {
              tunnel: w193 -> [w201] mode=indexing
              tunnel: [w202] -> w189 mode=indexing
              tunnel: w188 -> [w200]
              n68 = Unbundle By Name(w201) -> ("ID"=w198:string)
              n69 = Format Into String(format string="subject=\"%s\"", w198) -> (resulting string=w196:string)  [unwired: 2 in, 1 out]
              n70 = while {
                tunnel: w198 -> [_]
                shift-right: [w214] -> _
                shift-left: 0 ("offset past match") -> [w215]
                tunnel: w200 -> [w211]
                tunnel: w196 -> [w210]
                tunnel: [w204] -> w195
                tunnel: [w203] -> w194
                stop <- w207 stop-if-true
                n71 = Match Pattern(string=w211, regular expression="<element geometry=", offset (0)=w215) -> (after substring=w205:string, offset past match=w214:i32)  [unwired: 2 out]
                n72 = Match Pattern(string=w205, regular expression="[\\n\\r]") -> (before substring=w212:string)  [unwired: 1 in, 3 out]
                n73 = Empty String/Path?(string/path=w205) -> (empty?=w208:bool)
                n74 = Match Pattern(string=w212, regular expression=w210) -> (offset past match=w209:i32)  [unwired: 1 in, 3 out]
                n75 = Greater Or Equal To 0?(x=w209) -> (x >= 0?=w206:bool)
                n76 = Or(x=w208, y=w206) -> (x .or. y?=w207:bool)
                n77 = case shown="False" w206 {
                  tunnel: w205 -> [_ w225]
                  tunnel: [w217 w221] -> w204
                  tunnel: [w217 w218] -> w203
                  frame False {
                    w217 = -1 ("default (0 I32)")
                  }
                  frame True {
                    w219 = -1 ("default (0 I32)")
                    w223 = "[0-9]+" ("regular expression")
                    n78 = Match Pattern(string=w225, regular expression=w223) -> (match substring=w222:string, after substring=w224:string)  [unwired: 1 in, 2 out]
                    n79 = Match Pattern(string=w224, regular expression=w223) -> (match substring=w220:string)  [unwired: 1 in, 3 out]
                    n80 = Decimal String To Number(string=w222, default (0L)=w219) -> (number=w221:i32)  [unwired: 1 in, 1 out]
                    n81 = Decimal String To Number(string=w220, default (0L)=w219) -> (number=w218:i32)  [unwired: 1 in, 1 out]
                  }
                }
              }
              n82 = Bundle By Name(cluster=w201, "X"=w195, "Y"=w194) -> (w202:T9)
            }
            n83 = Bundle By Name(cluster=w192, "Classes"=w189) -> (w190:T17)
          }
          frame "GetClassAttributes" {
            # "<ownedAttribute xmi:type=\"uml:Property\" xmi:id=\"EAID_EC663448_03C2_4f90_B9CA_62EBF372B5D1\" name=\"Flow\" visibility=\"private\" isStatic=\"false\" isReadOnly=\"false\" isDerived=\"false\" isOrdered=\"false\" isUnique=\"true\" isDerivedUnion=\"false\">\n\t\t\t\t\t<lowerValue xmi:type=\"uml:LiteralInteger\" xmi:id=\"EAID_LI000001_03C2_4f90_B9CA_62EBF372B5D1\" value=\"1\"/>\n\t\t\t\t\t<upperValue xmi:type=\"uml:LiteralUnlimitedNatural\" xmi:id=\"EAID_LI000002_03C2_4f90_B9CA_62EBF372B5D1\" value=\"1\"/>\n\t\t\t\t\t<type xmi:idref=\"EAJava_DBL\"/>\n\t\t\t\t</ownedAttribute>"
            n84 = Unbundle By Name(w230) -> ("ClasseStrings"=w233:string[])
            n85 = for {
              tunnel: w233 -> [w241] mode=indexing
              tunnel: string[] ["xmi:id=\"", "name=\"", "visibility=\"", "<type xmi:idref=\"", "association=\""] -> [w238]
              shift-right: [w235] -> w229
              shift-left: cluster{T8[]}[] [] -> [w234]
              n86 = while {
                tunnel: w241 -> [w254]
                tunnel: w238 -> [w250]
                shift-right: [w247] -> _
                shift-left: 0 -> [w249]
                shift-right: [w243] -> w237
                shift-left: T8[] [] -> [w244]
                stop <- w242 continue-if-true
                n87 = Match Pattern(string=w254, regular expression="<ownedAttribute", offset (0)=w249) -> (after substring=w252:string, offset past match=w248:i32)  [unwired: 2 out]
                n88 = Match Pattern(string=w252, regular expression="</ownedAttribute>") -> (before substring=w245:string, offset past match=w246:i32)  [unwired: 1 in, 2 out]
                n89 = Greater Or Equal To 0?(x=w246) -> (x >= 0?=w242:bool)
                n90 = Add(x=w246, y=w248) -> (x+y=w247:i32)
                n91 = case shown="True" w242 {
                  tunnel: w250 -> [_ w270]
                  tunnel: w245 -> [_ w264]
                  tunnel: w244 -> [w255 w261]
                  tunnel: [w255 w260] -> w243
                  frame False {
                  }
                  frame True {
                    n92 = for {
                      tunnel: w270 -> [w280] mode=indexing
                      tunnel: w264 -> [w279]
                      tunnel: [w275] -> w265 mode=indexing
                      n93 = Match Pattern(string=w279, regular expression=w280) -> (after substring=w278:string)  [unwired: 1 in, 3 out]
                      n94 = Match Pattern(string=w278, regular expression="\"") -> (before substring=w276:string)  [unwired: 1 in, 3 out]
                      n95 = call <vilib>:"Unescape XML.vi"("XML String In"=w276) -> ("XML String Out"=w275:string)  [unwired: 9 in, 1 out]
                    }
                    n96 = Index Array(array=w265) -> (element #1=w268:string, element #2=w258:string, element #3=w267:string, element #4=w262:string, element #5=w257:string)  [unwired: 5 in]
                    n97 = Scan From String(input string=w267, default 1=T18."public" ("Visibility")) -> (output 1=w266:T18)  [unwired: 3 in, 3 out]
                    n98 = Empty String/Path?(string/path=w258) -> ()  [unwired: 1 out]
                    n99 = Bundle(cluster=T8 {"ID"="", "Name"="", "Visibility"=enum."invalid scope", "RefIdType"="", "AssRefId"=""} ("Attribute"), "ID"=w268, "Name"=w258, "Visibility"=w266, "RefIdType"=w262, "AssRefId"=w257) -> (w259:T8)
                    n100 = case shown="False" FALSE {
                      tunnel: w261 -> [w273 w274]
                      tunnel: [w272 w274] -> w260
                      tunnel: w259 -> [w271 _]
                      frame False {
                        n101 = Build Array (concatenate)(w273, w271) -> (w272:T8[])
                      }
                      frame True {
                      }
                    }
                  }
                }
              }
              n102 = Bundle(w237) -> (w236:cluster{T8[]})  [unwired: 1 in]
              n103 = Build Array (concatenate)(w234, w236) -> (w235:cluster{T8[]}[])
            }
            n104 = Bundle By Name(cluster=w230, "ClassAttributes"=w229) -> (w228:T17)
          }
          frame "GetClassMethods" {
            # "<ownedOperation xmi:id=\"EAID_10F4F595_2E67_4f8b_B085_F3130FD6B91C\" name=\"FlowSensorTest\" visibility=\"public\" concurrency=\"sequential\">\n\t\t\t\t\t<ownedParameter xmi:id=\"EAID_RT000000_2E67_4f8b_B085_F3130FD6B91C\" name=\"return\" direction=\"return\" type=\"EAJava_void\"/>\n\t\t\t\t</ownedOperation>"
            n105 = Unbundle By Name(w285) -> ("ClasseStrings"=w288:string[])
            n106 = for {
              tunnel: w288 -> [w296] mode=indexing
              tunnel: string[] ["xmi:id=\"", "name=\"", "visibility=\""] -> [w293]
              shift-right: [w290] -> w284
              shift-left: cluster{T7[]}[] [] -> [w289]
              n107 = while {
                tunnel: w296 -> [w309]
                tunnel: w293 -> [w305]
                shift-right: [w302] -> _
                shift-left: 0 -> [w304]
                shift-right: [w298] -> w292
                shift-left: T7[] [] -> [w299]
                stop <- w297 continue-if-true
                n108 = Match Pattern(string=w309, regular expression="<ownedOperation", offset (0)=w304) -> (after substring=w307:string, offset past match=w303:i32)  [unwired: 2 out]
                n109 = Match Pattern(string=w307, regular expression="</ownedOperation>") -> (before substring=w300:string, offset past match=w301:i32)  [unwired: 1 in, 2 out]
                n110 = Greater Or Equal To 0?(x=w301) -> (x >= 0?=w297:bool)
                n111 = Add(x=w301, y=w303) -> (x+y=w302:i32)
                n112 = case shown="True" w297 {
                  tunnel: w305 -> [_ w322]
                  tunnel: w300 -> [_ w315]
                  tunnel: w299 -> [w310 w313]
                  tunnel: [w310 w312] -> w298
                  frame False {
                  }
                  frame True {
                    n113 = for {
                      tunnel: w322 -> [w328] mode=indexing
                      tunnel: w315 -> [w327]
                      tunnel: [w323] -> w316 mode=indexing
                      n114 = Match Pattern(string=w327, regular expression=w328) -> (after substring=w326:string)  [unwired: 1 in, 3 out]
                      n115 = Match Pattern(string=w326, regular expression="\"") -> (before substring=w324:string)  [unwired: 1 in, 3 out]
                      n116 = call <vilib>:"Unescape XML.vi"("XML String In"=w324) -> ("XML String Out"=w323:string)  [unwired: 9 in, 1 out]
                    }
                    n117 = Index Array(array=w316) -> (element #1=w320:string, element #2=w319:string, element #3=w318:string)  [unwired: 4 in, 1 out]
                    n118 = Scan From String(input string=w318, default 1=T18."public" ("Visibility")) -> (output 1=w317:T18)  [unwired: 3 in, 3 out]
                    n119 = Bundle(cluster=T7 {"ID"="", "Name"="", "Visibility"=enum."invalid scope"} ("Attribute"), "ID"=w320, "Name"=w319, "Visibility"=w317) -> (w311:T7)
                    n120 = Build Array (concatenate)(w313, w311) -> (w312:T7[])
                  }
                }
              }
              n121 = Bundle(w292) -> (w291:cluster{T7[]})  [unwired: 1 in]
              n122 = Build Array (concatenate)(w289, w291) -> (w290:cluster{T7[]}[])
            }
            n123 = Bundle By Name(cluster=w285, "ClassMethods"=w284) -> (w283:T17)
          }
          frame "GetClassGeneralizations" {
            # "<links>\n\t\t\t\t\t<Generalization xmi:id=\"EAID_0DE68257_7B73_49de_8911_6A86EEA6B0BA\" start=\"EAID_C3DA8127_A723_4109_B2F4_88FBFDB77E9A\" end=\"EAID_9D25F9E0_C95B_4aa1_AC76_B051C1862941\"/>\n\t\t\t\t\t<Aggregation xmi:id=\"EAID_A6816E9D_1FF1_4b60_8E7A_E0ACE5709CF7\" start=\"EAID_C026E737_BCF9_4d6d_B726_90C39C0C8268\" end=\"EAID_9D25F9E0_C95B_4aa1_AC76_B051C1862941\"/>\n\t\t\t\t</links>"
            # "<generalization xmi:type=\"uml:Generalization\""
            # "<generalization xmi:type=\"uml:Generalization\" xmi:id=\"EAID_D3817FF1_0384_46a8_B09D_8F9D9E807829\" general=\"EAID_BDBB4C97_A1E7_4ecc_B5E2_52D4EA971126\"/>"
            n124 = Unbundle By Name(w333) -> ("ClasseStrings"=w336:string[])
            n125 = for {
              tunnel: w336 -> [w345] mode=indexing
              tunnel: string[] ["xmi:id=\"", "general=\""] -> [w343]
              shift-right: [w340] -> w332
              shift-left: cluster{"Genarilization":T3[]}[] [] -> [w339]
              n126 = while {
                tunnel: w345 -> [w358]
                tunnel: w343 -> [w355]
                shift-right: [w352] -> _
                shift-left: 0 -> [w354]
                shift-right: [w348] -> w342
                shift-left: T3[] [] ("Genarilization") -> [w349]
                tunnel: "<generalization xmi:type=\"uml:Generalization\"" ("regular expression") -> [w346]
                stop <- w347 continue-if-true
                n127 = Match Pattern(string=w358, regular expression=w346, offset (0)=w354) -> (after substring=w357:string, offset past match=w353:i32)  [unwired: 2 out]
                n128 = Match Pattern(string=w357, regular expression=">") -> (before substring=w350:string, offset past match=w351:i32)  [unwired: 1 in, 2 out]
                n129 = Greater Or Equal To 0?(x=w351) -> (x >= 0?=w347:bool)
                n130 = Add(x=w351, y=w353) -> (x+y=w352:i32)
                n131 = case shown="True" w347 {
                  tunnel: w355 -> [_ w368]
                  tunnel: w350 -> [_ w364]
                  tunnel: w349 -> [w359 w363]
                  tunnel: [w359 w362] -> w348
                  frame False {
                  }
                  frame True {
                    n132 = for {
                      tunnel: w368 -> [w374] mode=indexing
                      tunnel: w364 -> [w373]
                      tunnel: [w369] -> w365 mode=indexing
                      n133 = Match Pattern(string=w373, regular expression=w374) -> (after substring=w372:string)  [unwired: 1 in, 3 out]
                      n134 = Match Pattern(string=w372, regular expression="\"") -> (before substring=w370:string)  [unwired: 1 in, 3 out]
                      n135 = call <vilib>:"Unescape XML.vi"("XML String In"=w370) -> ("XML String Out"=w369:string)  [unwired: 9 in, 1 out]
                    }
                    n136 = Index Array(array=w365) -> (element #1=w367:string, element #2=w366:string)  [unwired: 4 in, 2 out]
                    n137 = Bundle(cluster=T3 {"ID"="", "ClassID"=""} ("Association"), "ID"=w367, "ClassID"=w366) -> (w361:T3)
                    n138 = Build Array (concatenate)(w363, w361) -> (w362:T3[])
                  }
                }
              }
              n139 = Bundle("Genarilization"=w342) -> (w341:cluster{"Genarilization":T3[]})  [unwired: 1 in]
              n140 = Build Array (concatenate)(w339, w341) -> (w340:cluster{"Genarilization":T3[]}[])
            }
            n141 = Bundle By Name(cluster=w333, "ClassInheritance"=w332) -> (w331:T17)
          }
          frame "GetTypes" {
            # "<packagedElement xmi:type=\"uml:Package\" xmi:id=\"EAJavaTypesPackage\" name=\"EA_Java_Types_Package\" visibility=\"public\">\n\t\t\t\t\t<packagedElement xmi:type=\"uml:PrimitiveType\" xmi:id=\"EAJava_DBL\" name=\"DBL\" visibility=\"public\"/>\n\t\t\t\t\t<packagedElement xmi:type=\"uml:PrimitiveType\" xmi:id=\"EAJava_TempSensor\" name=\"TempSensor\" visibility=\"public\"/>\n\t\t\t\t\t<packagedElement xmi:type=\"uml:PrimitiveType\" xmi:id=\"EAJava_void\" name=\"void\" visibility=\"public\"/>\n\t\t\t\t\t<packagedElement xmi:type=\"uml:PrimitiveType\" xmi:id=\"EAJava_UINT8\" name=\"UINT8\" visibility=\"public\"/>\n\t\t\t\t\t<packagedElement xmi:type=\"uml:PrimitiveType\" xmi:id=\"EAJava_Device__\" name=\"Device[]\" visibility=\"public\"/>\n\t\t\t\t\t<packagedElement xmi:type=\"uml:PrimitiveType\" xmi:id=\"EAJava_RefNum\" name=\"RefNum\" visibility=\"public\"/>\n\t\t\t\t</packagedElement>"
            n142 = Unbundle By Name(w384) -> ("text"=w386:string, "ClassAttributes"=w380:cluster{T8[]}[])
            n143 = for {
              tunnel: w380 -> [w418] mode=indexing
              shift-right: [w416] -> w378
              shift-left: string[] [] -> [w415]
              n144 = Unbundle(w418) -> (w417:T8[])
              n145 = for {
                tunnel: w417 -> [w422] mode=indexing
                shift-right: [w419] -> w416
                shift-left: w415 -> [w421]
                n146 = Unbundle(w422) -> ("RefIdType"=w420:string)  [unwired: 4 out]
                n147 = Build Array (concatenate)(w421, w420) -> (w419:string[])
              }
            }
            n148 = for {
              tunnel: w386 -> [w398]
              tunnel: string[] ["name=\""] -> [w395]
              shift-right: [w393] -> w376
              shift-left: T6[] [] -> [w394]
              tunnel: w378 -> [w389] mode=indexing
              tunnel: "xmi:id=\"%s" -> [w388]
              n149 = Format Into String(format string=w388, w389) -> (resulting string=w391:string)  [unwired: 2 in, 1 out]
              n150 = Match Pattern(string=w398, regular expression=w391) -> (after substring=w397:string)  [unwired: 1 in, 3 out]
              n151 = Match Pattern(string=w397, regular expression="\"") -> (after substring=w387:string, offset past match=w390:i32)  [unwired: 1 in, 2 out]
              n152 = Greater Or Equal To 0?(x=w390) -> (x >= 0?=w392:bool)
              n153 = case shown="True" w392 {
                tunnel: w395 -> [_ w408]
                tunnel: w387 -> [_ w406]
                tunnel: w394 -> [w399 w405]
                tunnel: [w399 w404] -> w393
                tunnel: w389 -> [_ w400]
                frame False {
                }
                frame True {
                  n154 = for {
                    tunnel: w408 -> [w414] mode=indexing
                    tunnel: w406 -> [w413]
                    tunnel: [w409] -> w407 mode=indexing
                    n155 = Match Pattern(string=w413, regular expression=w414) -> (after substring=w412:string)  [unwired: 1 in, 3 out]
                    n156 = Match Pattern(string=w412, regular expression="\"") -> (before substring=w410:string)  [unwired: 1 in, 3 out]
                    n157 = call <vilib>:"Unescape XML.vi"("XML String In"=w410) -> ("XML String Out"=w409:string)  [unwired: 9 in, 1 out]
                  }
                  n158 = Index Array(array=w407) -> (element #1=w401:string)  [unwired: 2 in, 1 out]
                  n159 = Bundle(cluster=T6 {"ID"="", "Name"=""} ("Attribute"), "ID"=w400, "Name"=w401) -> (w403:T6)
                  n160 = Build Array (concatenate)(w405, w403) -> (w404:T6[])
                }
              }
            }
            n161 = Bundle By Name(cluster=w384, "Types"=w376) -> (w383:T17)
          }
          frame "FindAssociations" {
            # "<memberEnd xmi:idref=\"EAID_dst1490FC_8515_4843_A058_F8B338EB0930\"/>\n\t\t\t\t\t<memberEnd xmi:idref=\"EAID_src1490FC_8515_4843_A058_F8B338EB0930\"/>\n\t\t\t\t\t<ownedEnd xmi:type=\"uml:Property\" xmi:id=\"EAID_src1490FC_8515_4843_A058_F8B338EB0930\" visibility=\"public\" association=\"EAID_DE1490FC_8515_4843_A058_F8B338EB0930\" isStatic=\"false\" isReadOnly=\"false\" isDerived=\"false\" isOrdered=\"false\" isUnique=\"true\" isDerivedUnion=\"false\" aggregation=\"shared\">\n\t\t\t\t\t\t<type xmi:idref=\"EAID_C026E737_BCF9_4d6d_B726_90C39C0C8268\"/>\n\t\t\t\t\t</ownedEnd>"
            # "<packagedElement xmi:type=\"uml:Association\" xmi:id=\"EAID_F3B66838_A6D7_4f82_9283_F2214000E925\" visibility=\"public\">\n\t\t\t\t\t<memberEnd xmi:idref=\"EAID_dstB66838_A6D7_4f82_9283_F2214000E925\"/>\n\t\t\t\t\t<ownedEnd xmi:type=\"uml:Property\" xmi:id=\"EAID_dstB66838_A6D7_4f82_9283_F2214000E925\" visibility=\"public\" association=\"EAID_F3B66838_A6D7_4f82_9283_F2214000E925\" isStatic=\"false\" isReadOnly=\"false\" isDerived=\"false\" isOrdered=\"false\" isUnique=\"true\" isDerivedUnion=\"false\" aggregation=\"none\">\n\t\t\t\t\t\t<type xmi:idref=\"EAID_BDBB4C97_A1E7_4ecc_B5E2_52D4EA971126\"/>\n\t\t\t\t\t</ownedEnd>\n\t\t\t\t\t<memberEnd xmi:idref=\"EAID_srcB66838_A6D7_4f82_9283_F2214000E925\"/>\n\t\t\t\t\t<ownedEnd xmi:type=\"uml:Property\" xmi:id=\"EAID_srcB66838_A6D7_4f82_9283_F2214000E925\" visibility=\"public\" association=\"EAID_F3B66838_A6D7_4f82_9283_F2214000E925\" isStatic=\"false\" isReadOnly=\"false\" isDerived=\"false\" isOrdered=\"false\" isUnique=\"true\" isDerivedUnion=\"false\" aggregation=\"none\">\n\t\t\t\t\t\t<type xmi:idref=\"EAID_08B756DE_5C06_4edc_9F0A_D17F3D5FFCDA\"/>\n\t\t\t\t\t</ownedEnd>\n\t\t\t\t</packagedElement>"
            n162 = Unbundle By Name(w423) -> ("text"=w425:string)
            n163 = disable-structure shown="Enabled" {
              disable-tunnel: [w433 w451] -> w426
              disable-tunnel: w425 -> [w432 _]
              disable-tunnel: w423 -> [w431 w451]
              frame Enabled {
                (unwired) string[] []
                n164 = while {
                  tunnel: w432 -> [w445]
                  shift-right: [w434] -> _
                  shift-left: 0 ("offset past match") -> [w439]
                  shift-right: [w438] -> w428
                  shift-left: T4[] [] -> [w437]
                  stop <- w440 continue-if-true
                  n165 = Match Pattern(string=w445, regular expression="<packagedElement xmi:type=\"uml:Association\"", offset (0)=w439) -> (after substring=w443:string, offset past match=w436:i32)  [unwired: 2 out]
                  n166 = Match Pattern(string=w443, regular expression="</packagedElement>") -> (before substring=w441:string, offset past match=w435:i32)  [unwired: 1 in, 2 out]
                  n167 = Greater Or Equal To 0?(x=w435) -> (x >= 0?=w440:bool)
                  n168 = Add(x=w435, y=w436) -> (x+y=w434:i32)
                  n169 = case shown="True" w440 {
                    tunnel: w441 -> [_ w450]
                    tunnel: w437 -> [w446 w448]
                    tunnel: [w446 w449] -> w438
                    frame False {
                    }
                    frame True {
                      n170 = call <resource>:"UMLEditor_ReadXmiFile_AnalyseAssText.vi"("text"=w450) -> ("Association"=w447:T4)
                      n171 = Build Array (concatenate)(w448, w447) -> (w449:T4[])
                    }
                  }
                }
                n172 = Bundle By Name(cluster=w431, "Associations"=w428) -> (w433:T17)
              }
              frame Disabled {
              }
            }
          }
          frame "UpdateClassInfo" {
            n173 = Unbundle By Name(w461) -> ("ClassLinks"=→"ClassLinks":cluster{T1[]}[], "Associations"=→"Associations":T4[], "Classes"=w459:T9[], "ClassAttributes"=w467:cluster{T8[]}[], "ClassMethods"=w468:cluster{T7[]}[], "Types"=w465:T6[], "ClassInheritance"=w457:cluster{"Genarilization":T3[]}[])
            "Classes" <- w459
            "ClassAttributes" <- w467
            "ClassMethods" <- w468
            "Types" <- w465
            "ClassInheritance" <- w457
            n174 = for {
              tunnel: w465 -> [w478] mode=indexing
              tunnel: [w477] -> w464 mode=indexing
              tunnel: [w476] -> w463 mode=indexing
              n175 = Unbundle By Name(w478) -> ("ID"=w477:string, "Name"=w476:string)
            }
            n176 = for {
              tunnel: [w472] -> w458 mode=indexing
              tunnel: w459 -> [w475] mode=indexing
              tunnel: [w474] -> w456 mode=indexing
              tunnel: [w471] -> w452 mode=indexing
              n177 = Unbundle By Name(w475) -> ("ID"=w474:string, "Name"=w472:string)
              n178 = Bundle(cluster=T19 {"ClassNamn"="", "ClassPath"=path "", "InterfaceClass"=FALSE} ("Cluster"), "ClassNamn"=w472) -> (w471:T19)  [unwired: 2 in]
            }
            n179 = for {
              tunnel: w459 -> [w524] mode=indexing
              tunnel: w468 -> [w522] mode=indexing
              tunnel: w467 -> [w519] mode=indexing
              tunnel: w464 -> [w515]
              tunnel: w463 -> [w514]
              tunnel: [w513] -> w462 mode=indexing
              tunnel: w458 -> [w504]
              tunnel: w457 -> [w510] mode=indexing
              tunnel: w456 -> [w506]
              tunnel: [w488] -> w455 mode=indexing
              tunnel: w454 -> [w480]
              tunnel: w452 -> [w479]
              n180 = Unbundle(w519) -> (w518:T8[])
              n181 = Unbundle(w510) -> ("Genarilization"=w509:T3[])
              n182 = Unbundle By Name(w524) -> ("Name"=w497:string, "Stereotype"=w492:string, "Description"=w491:string, "X"=w490:i32, "Y"=w489:i32)
              n183 = Unbundle(w522) -> (w521:T7[])
              n184 = Index Array(array=w509) -> (element=w508:T3)  [unwired: 1 in]
              n185 = for {
                tunnel: w518 -> [w535] mode=indexing
                tunnel: T11 {"name"="", "type"=enum."UINT8", "dimension"=0, "typeName"="", "typePath"=path "", "visibility"=enum."Public"} ("attributeInfoType") -> [w534]
                shift-right: [w529] -> w512
                shift-left: T11[] [] -> [w530]
                tunnel: w515 -> [w528]
                tunnel: w514 -> [w526]
                tunnel: w504 -> [_]
                tunnel: w479 -> [w525]
                n186 = Unbundle By Name(w535) -> ("Name"=w532:string, "Visibility"=w533:T18, "RefIdType"=w527:string)  [unwired: 1 out]
                n187 = Empty String/Path?(string/path=w532) -> (empty?=w531:bool)
                n188 = case shown="False" w531 {
                  tunnel: w534 -> [w551 _]
                  tunnel: w533 -> [w550 _]
                  tunnel: w532 -> [w548 _]
                  tunnel: w530 -> [w547 w555]
                  tunnel: [w546 w555] -> w529
                  tunnel: w528 -> [w544 _]
                  tunnel: w527 -> [w543 _]
                  tunnel: w526 -> [w542 _]
                  tunnel: w525 -> [w536 _]
                  frame False {
                    n189 = Search 1D Array(1D array=w544, element=w543) -> (index of element=w541:i32)  [unwired: 1 in]
                    n190 = Index Array(array=w542, index=w541) -> (element=w540:string)
                    n191 = case shown="\"protected\"" w550 {
                      tunnel: [CommonVIs_VisibilityType."Private" ("Enum") CommonVIs_VisibilityType."Public" ("Enum") CommonVIs_VisibilityType."Protected" ("Enum")] -> w549
                      frame "private" {
                      }
                      frame "public", Default {
                      }
                      frame "protected" {
                      }
                    }
                    n192 = call <resource>:"CommonVIs_GetDatatypeFromString.vi"("String"=w540, "Classes"=w536) -> ("AttributeDataType"=w539:T12, "ArrayDimensions"=w538:i32, "DataTypeAsString(Array,default values removed)"=w537:string)  [unwired: 9 in, 2 out]
                    n193 = Bundle By Name(cluster=w551, "name"=w548, "type"=w539, "dimension"=w538, "typeName"=w537, "visibility"=w549) -> (w545:T11)
                    n194 = Build Array (concatenate)(w547, w545) -> (w546:T11[])
                  }
                  frame True {
                  }
                }
              }
              n195 = for {
                tunnel: [w559] -> w523 mode=indexing
                tunnel: w521 -> [w558] mode=indexing
                tunnel: [w557] -> w520 mode=indexing
                n196 = Unbundle By Name(w558) -> ("Name"=w557:string, "Visibility"=w556:T18)
                n197 = case shown="\"protected\"" w556 {
                  tunnel: [CommonVIs_VisibilityType."Private" ("Enum") CommonVIs_VisibilityType."Public" ("Enum") CommonVIs_VisibilityType."Protected" ("Enum")] -> w559
                  frame "private" {
                  }
                  frame "public", Default {
                  }
                  frame "protected" {
                  }
                }
              }
              n198 = Bundle("X"=w490, "Y"=w489) -> (w488:cluster{"X":i32, "Y":i32})  [unwired: 1 in]
              n199 = Concatenate Strings(w497, ".lvclass" ("string")) -> (w496:string)
              n200 = Unbundle By Name(w508) -> ("ClassID"=w507:string)
              n201 = String To Path(string=w496) -> (path=w483:path)
              n202 = Search 1D Array(1D array=w506, element=w507) -> (index of element=w505:i32)  [unwired: 1 in]
              n203 = Build Path(base path=w480, name or relative path=w483) -> (appended path=w484:path)
              n204 = Index Array(array=w504, index=w505) -> (element=w485:string)
              n205 = Empty String/Path?(string/path=w485) -> (empty?=w503:bool)
              n206 = Concatenate Strings(w485, ".lvclass" ("string")) -> (w486:string)
              n207 = String To Path(string=w486) -> (path=w482:path)
              n208 = Not(x=w503) -> (.not. x?=w502:bool)
              n209 = Build Path(base path=w480, name or relative path=w482) -> (appended path=w481:path)
              n210 = Format Into String(format string="<<%s>>\n%s", w492, w491) -> (resulting string=w494:string)  [unwired: 2 in, 1 out]
              n211 = Build Array(w481) -> (w501:path[])
              n212 = call <vilib>:"Trim Whitespace.vi"("string"=w494) -> ("trimmed string"=w493:string)  [unwired: 1 in]
              n213 = Select(t=w501, s=w502, f=path[] []) -> (s? t:f=w499:path[])
              n214 = Bundle By Name(cluster=T14 {"classPath"=path "", "inherits"=FALSE, "baseClasses"=[], "compAggClasses"=[], "noOfCompObj"=[], "aggClasses"=[], "noOfAgg"=[], "depClasses"=[], "methods"=[], "methodPuplic"=[], "objectAttrib"=[], "classAttrib"=[], "ClassDesc"="", "DependencyDetails"=[], "Interface"=FALSE, "ParentInterfaces"=[]} ("classInfo"), "ClassDesc"=w493, "classPath"=w484, "methods"=w520, "methodPuplic"=w523, "objectAttrib"=w512, "inherits"=w502, "baseClasses"=w499) -> (w513:T14)
            }
            n215 = Bundle By Name(cluster=w461, "classInfos"=w462, "Positions"=w455) -> (w460:T17)
          }
          frame "UpdateClassAssosications" {
            n216 = Unbundle By Name(w564) -> ("classInfos"=w576:T14[], "Classes"=w573:T9[])
            n217 = Unbundle By Name(w564) -> ("ClassLinks"=w567:cluster{T1[]}[], "Associations"=w566:T4[])
            n218 = Unbundle By Name(w564) -> ("ClassAttributes"=w563:cluster{T8[]}[])
            n219 = for {
              tunnel: w566 -> [w740] mode=indexing
              tunnel: [w739] -> w565 mode=indexing
              n220 = Unbundle By Name(w740) -> ("ID"=w739:string)
            }
            n221 = for {
              tunnel: [w743] -> w570 mode=indexing
              tunnel: w573 -> [w742] mode=indexing
              tunnel: [w741] -> w571 mode=indexing
              n222 = Unbundle By Name(w742) -> ("ID"=w741:string, "Name"=w743:string)
            }
            n223 = disable-structure shown="Enabled" {
              disable-tunnel: w576 -> [w582 w655]
              disable-tunnel: [w581 w654] -> w572
              disable-tunnel: w566 -> [w580 w650]
              disable-tunnel: w571 -> [w579 w649]
              disable-tunnel: w570 -> [w578 w648]
              disable-tunnel: w569 -> [w577 w653]
              disable-tunnel: w567 -> [_ w652]
              disable-tunnel: w565 -> [_ w651]
              disable-tunnel: w563 -> [_ w647]
              frame Disabled {
                n224 = for {
                  shift-right: [w600] -> w581
                  shift-left: w582 -> [w601]
                  tunnel: w580 -> [w599] mode=indexing
                  tunnel: w579 -> [w598]
                  tunnel: w578 -> [w597]
                  tunnel: w577 -> [w594]
                  tunnel: _ -> [w587]
                  n225 = Unbundle By Name(w599) -> ("IdRef1"=w588:string, "IdRef1Type"=w584:T5, "IdRef2"=w586:string)  [unwired: 1 out]
                  n226 = Search 1D Array(1D array=w598, element=w588) -> (index of element=w590:i32)  [unwired: 1 in]
                  n227 = Search 1D Array(1D array=w598, element=w586) -> (index of element=w585:i32)  [unwired: 1 in]
                  n228 = case shown="-1" w590 {
                    selector: w590 -> [w615 _]
                    tunnel: [w615 w616] -> w589
                    tunnel: w587 -> [_ w621]
                    tunnel: w588 -> [_ w620]
                    frame 0, Default {
                    }
                    frame -1 {
                      n229 = for {
                        tunnel: w621 -> [w627] mode=indexing
                        tunnel: w620 -> [w625]
                        tunnel: [w623] -> w619
                        tunnel: [w622] -> w618
                        i -> [w622]
                        stop <- w623 stop-if-true
                        n230 = Unbundle(w627) -> (w626)
                        n231 = Search 1D Array(1D array=w626, element=w625) -> (index of element=w624:i32)  [unwired: 1 in]
                        n232 = Greater Or Equal To 0?(x=w624) -> (x >= 0?=w623:bool)
                      }
                      n233 = Select(t=w618, s=w619, f=-1) -> (s? t:f=w616:i32)
                    }
                  }
                  n234 = case shown="-1" w585 {
                    selector: w585 -> [w602 _]
                    tunnel: [w602 w603] -> w583
                    tunnel: w587 -> [_ w608]
                    tunnel: w586 -> [_ w607]
                    frame 0, Default {
                    }
                    frame -1 {
                      n235 = for {
                        tunnel: w608 -> [w614] mode=indexing
                        tunnel: w607 -> [w612]
                        tunnel: [w610] -> w606
                        tunnel: [w609] -> w605
                        i -> [w609]
                        stop <- w610 stop-if-true
                        n236 = Unbundle(w614) -> (w613)
                        n237 = Search 1D Array(1D array=w613, element=w612) -> (index of element=w611:i32)  [unwired: 1 in]
                        n238 = Greater Or Equal To 0?(x=w611) -> (x >= 0?=w610:bool)
                      }
                      n239 = Select(t=w605, s=w606, f=-1) -> (s? t:f=w603:i32)
                    }
                  }
                  n240 = Index Array(array=w597, index=w583) -> (element=w592:string)
                  n241 = Concatenate Strings(w592, ".lvclass" ("string")) -> (w596:string)
                  n242 = String To Path(string=w596) -> (path=w595:path)
                  n243 = Build Path(base path=w594, name or relative path=w595) -> (appended path=w591:path)
                  n244 = in-place {
                    in-place-border: w591 -> [w629]
                    in-place-border: w584 -> [w628]
                    n245 = in-place-array #1(w601, w589) -> (w630:T14)
                    n246 = case shown="Default" w628 {
                      tunnel: [w636 w641 w646] -> w631
                      tunnel: w630 -> [w635 w640 w645]
                      tunnel: w629 -> [w632 w637 w642]
                      frame "Shared" {
                        n247 = Unbundle By Name(w635) -> ("aggClasses"=w634:path[])
                        n248 = Build Array (concatenate)(w634, w632) -> (w633:path[])
                        n249 = Bundle By Name(cluster=w635, "aggClasses"=w633) -> (w636:T14)
                      }
                      frame "Composite" {
                        n250 = Unbundle By Name(w640) -> ("compAggClasses"=w639:path[])
                        n251 = Build Array (concatenate)(w639, w637) -> (w638:path[])
                        n252 = Bundle By Name(cluster=w640, "compAggClasses"=w638) -> (w641:T14)
                      }
                      frame Default {
                        n253 = Unbundle By Name(w645) -> ("depClasses"=w644:path[])
                        n254 = Build Array (concatenate)(w644, w642) -> (w643:path[])
                        n255 = Bundle By Name(cluster=w645, "depClasses"=w643) -> (w646:T14)
                      }
                    }
                    n256 = in-place-array #1(w631) -> (w600:T14[])  [unwired: 1 out]
                  }
                }
              }
              frame Enabled {
                n257 = for {
                  tunnel: w655 -> [w667] mode=indexing
                  tunnel: [w666] -> w654 mode=indexing
                  tunnel: w653 -> [w665]
                  tunnel: w652 -> [w664] mode=indexing
                  tunnel: w649 -> [w662] mode=indexing
                  tunnel: w651 -> [w661]
                  tunnel: w650 -> [w660]
                  tunnel: w649 -> [w659]
                  tunnel: w648 -> [w658]
                  tunnel: w647 -> [w657] mode=indexing
                  # "If A has Ass Attribute link to B, then A is part of B, i.e. B is Aggregating A"
                  n258 = Unbundle(w664) -> (w663:T1[])
                  n259 = Unbundle(w657) -> (w656:T8[])
                  n260 = for {
                    tunnel: w665 -> [w702]
                    tunnel: w663 -> [w701] mode=indexing
                    shift-right: [w703] -> w666
                    shift-left: w667 -> [w704]
                    tunnel: w662 -> [w700]
                    tunnel: w661 -> [w694]
                    tunnel: w660 -> [w692]
                    tunnel: w659 -> [w683]
                    tunnel: w658 -> [w681]
                    tunnel: w656 -> [w677]
                    w687 = UMLEditor_ReadXmiFile_AssType."Composite" ("IdRef1Type")
                    # "Steps:\n-Find Ass with the Link ID\n-Check which class ass this Ass in it's attribute\n-If this class has it's in it's attribute, this class should not add the Association."
                    # "Only Add Ass if this class Aggregates the other class"
                    n261 = Unbundle By Name(w701) -> ("ID"=w693:string, "Start"=w697:string, "End"=w698:string, "Linktype"=w696:T2)
                    n262 = for {
                      tunnel: w677 -> [w706] mode=indexing
                      tunnel: [w705] -> w668 mode=indexing
                      n263 = Unbundle By Name(w706) -> ("ID"=w705:string)  [unwired: 4 out]
                    }
                    n264 = Search 1D Array(1D array=w694, element=w693) -> (index of element=w691:i32)  [unwired: 1 in]
                    n265 = Equal?(x=w700, y=w697) -> (x = y?=w699:bool)
                    n266 = Index Array(array=w692, index=w691) -> (element=w690:T4)
                    n267 = Unbundle By Name(w690) -> ("IdRef1Type"=w689:T5, "IdRef2Type"=w688:T5, "IdRef1"=w676:string, "IdRef2"=w675:string)
                    n268 = Select(t=w698, s=w699, f=w697) -> (s? t:f=w682:string)
                    n269 = Search 1D Array(1D array=w683, element=w682) -> (index of element=w680:i32)  [unwired: 1 in]
                    n270 = Search 1D Array(1D array=w668, element=w675) -> (index of element=w673:i32)  [unwired: 1 in]
                    n271 = Search 1D Array(1D array=w668, element=w676) -> (index of element=w674:i32)  [unwired: 1 in]
                    n272 = Greater Or Equal To 0?(x=w674) -> (x >= 0?=w672:bool)
                    n273 = Greater Or Equal To 0?(x=w673) -> (x >= 0?=w671:bool)
                    n274 = Index Array(array=w681, index=w680) -> (element=w679:string)
                    n275 = Equal?(x=w689, y=w687) -> (x = y?=w685:bool)
                    n276 = Or(x=w672, y=w671) -> (x .or. y?=w670:bool)
                    n277 = Equal?(x=w688, y=w687) -> (x = y?=w686:bool)
                    n278 = Not(x=w670) -> (.not. x?=w669:bool)
                    n279 = Or(x=w685, y=w686) -> (x .or. y?=w684:bool)
                    n280 = case shown="\"Aggregation\"" w696 {
                      tunnel: [UMLEditor_ReadXmiFile_AssType."None" ("IdRef1Type") w738] -> w695
                      tunnel: w684 -> [_ w735]
                      tunnel: [TRUE w734] -> w678
                      tunnel: w669 -> [_ w734]
                      frame "Association", Default {
                      }
                      frame "Aggregation" {
                        n281 = Select(t=UMLEditor_ReadXmiFile_AssType."Composite" ("IdRef1Type"), s=w735, f=UMLEditor_ReadXmiFile_AssType."Shared" ("IdRef1Type")) -> (s? t:f=w738:T5)
                      }
                    }
                    n282 = case shown="False" w678 {
                      tunnel: w704 -> [w707 w716]
                      tunnel: [w707 w715] -> w703
                      tunnel: w702 -> [_ w710]
                      tunnel: w695 -> [_ w709]
                      tunnel: w679 -> [_ w708]
                      frame False {
                      }
                      frame True {
                        n283 = Concatenate Strings(w708, ".lvclass" ("string")) -> (w714:string)
                        n284 = String To Path(string=w714) -> (path=w713:path)
                        n285 = Build Path(base path=w710, name or relative path=w713) -> (appended path=w711:path)
                        n286 = case shown="\"Shared\"" w709 {
                          tunnel: [w721 w726 w731] -> w715
                          tunnel: w716 -> [w720 w725 w730]
                          tunnel: w711 -> [w717 w722 w727]
                          frame "Shared" {
                            n287 = Unbundle By Name(w720) -> ("aggClasses"=w719:path[])
                            n288 = Build Array (concatenate)(w719, w717) -> (w718:path[])
                            n289 = Bundle By Name(cluster=w720, "aggClasses"=w718) -> (w721:T14)
                          }
                          frame "Composite" {
                            n290 = Unbundle By Name(w725) -> ("compAggClasses"=w724:path[])
                            n291 = Build Array (concatenate)(w724, w722) -> (w723:path[])
                            n292 = Bundle By Name(cluster=w725, "compAggClasses"=w723) -> (w726:T14)
                          }
                          frame Default {
                            n293 = Unbundle By Name(w730) -> ("depClasses"=w729:path[])
                            n294 = Build Array (concatenate)(w729, w727) -> (w728:path[])
                            n295 = Bundle By Name(cluster=w730, "depClasses"=w728) -> (w731:T14)
                          }
                        }
                      }
                    }
                  }
                }
              }
            }
            n296 = Bundle By Name(cluster=w564, "classInfos"=w572) -> (w575:T17)
          }
          frame "Error", Default {
          }
        }
        n297 = Unbundle By Name(w41) -> ("status"=w37:bool)
        n298 = Equal?(x=w40, y="Exit") -> (x = y?=w38:bool)
        n299 = Or(x=w38, y=w37) -> (x .or. y?=w36:bool)
      }
    }
    frame Error {
    }
  }
  n300 = Unbundle By Name(w18) -> ("TypeDefs"=w13:T10[], "classInfos"=w12:T14[], "VIRef"=w17:refnum<vi>[], "Positions"=→"Positions":cluster{"X":i32, "Y":i32}[])
  n301 = call <resource>:"Error_ClearError.vi"("codes"=i32[] [6100, 7000], "error in (no error)"=w16) -> ("Cleared?"=w14:bool, "error out"=→"error out":errorcluster)  [unwired: 3 in, 13 out]
  n302 = call <resource>:"Common_ ViCacheMemory.vi"("ViRef-Array"=w17) -> ()  [unwired: 3 in, 16 out]
  n303 = case shown="True" w14 {
    tunnel: w13 -> [w749 _]
    tunnel: w12 -> [w748 _]
    tunnel: [w749 _] -> w11
    tunnel: [w748 _] -> w6
    frame False {
    }
    frame True {
    }
  }
  "classInfos" <- w6
  "TypeDefs" <- w11
